vi "Demo Main.vi"() -> ()   [LabVIEW 2022 SP3]
uses:
  Logo.ctl
  C:/Users/Public/OneDrive/Desktop/PMT program/SampleCodeLabView/Kinesis_with_LabVIEW_Examples_LV12 - v3/Thorlabs.MotionControl.Controls.dll
  Kinesis_with_LabVIEW_Examples_LV12 - v3/Thorlabs.MotionControl.Controls.dll
  <vilib>/Utility/file.llb/Write Delimited Spreadsheet (string).vi
  <vilib>/Utility/file.llb/Write Delimited Spreadsheet (I64).vi
  <vilib>/Utility/file.llb/Write Delimited Spreadsheet (DBL).vi
  C:/Users/Public/OneDrive/Desktop/PMT program/SampleCodeLabView/Kinesis_with_LabVIEW_Examples_LV12 - v3/ThorLabs.MotionControl.KCube.DCServoCLI.dll
  Kinesis_with_LabVIEW_Examples_LV12 - v3/ThorLabs.MotionControl.KCube.DCServoCLI.dll
  <vilib>/Analysis/NI_AALBase.lvlib
panel:
  in  "SP 2":i32 caption="Start Position 2 \n Set Data\n(degrees)"
  out "SPD 2":i32 caption="Start Position 2\nRead Data"
  in  "second motor T/F":bool=TRUE
  out "PC 2":i32 caption="Current \nPosition 2"
  in  "Motor Controller\nSerialNumber 2":string="27260805"
  in  "KCubeDCServoControl 2":refnum<k24>(container)
  out "Polar Plot":picture
  in  "Wait to Start (ms)":i32
  in  "Laser Power (mW)":string="sample"
  in  "Sample Name":string="sample"
  in  "Save All Gate Data":bool
  out "ESD":i32=10000 caption="Steps\nAdded/Removed"
  in  "ES":i32 caption="Add /Remove \nSteps"
  out "Sweep Graph":u32[](graph)
  out "SM":i32 caption="Sweep\nMean"
  out "SN":i32 caption="Current Sweep Iteration"
  out "SND":i32 caption="Total No. of Sweeps"
  in  "Auto-Sweep":bool
  in  "P8":bool
  out "PC":i32 caption="Current \nPosition"
  out "WTD":i32=10000 caption="Wait Time (ms)\nRead Data"
  out "EPD":i32 caption="End Position\nRead Data"
  out "SPD":i32 caption="Start Position\nRead Data"
  out "SSD":i32 caption="Step Size\nRead Data"
  in  "SP":i32 caption="Start Position (degrees)\n Set Data"
  in  "WT":i32=5000 caption="Wait Time (ms)\n Set Data"
  in  "EP":i32 caption="End Position (degrees)\n Set Data"
  in  "P7":bool
  in  "SS":i32=10 caption="Step Size (degrees)\nSet Data"
  in  "Motor Controller\nSerialNumber":string="27261255"
  in  "KCubeDCServoControl":refnum<k24>(container)
  in  "Export":bool
  out "DB":u32[](array[numeric])
  out "OVL":bool caption="LED ON : Over Rang Data"
  out "OLD":i32
  out "GN":i32 caption="Gate Number"
  in  "Correction":bool=TRUE
  in  "Logo":T1
  out "Graph":u32[](graph)
  in  "Stop":bool
  in  "Start":bool
  in  "P6":bool
  out "RND":i32 caption="Read Number\nRead Data"
  in  "P5":bool
  in  "RN":i32=40 caption="Read Number\nSet Data"
  out "PowerD":i32 caption="Power\nRead Data"
  out "ITD":i32 caption="Internal Time\nRead Data"
  in  "P4":bool
  in  "P3":bool
  in  "IT":i32=100 caption="Internal Time\nSet Data"
  in  "P2":bool
  out "Handle Number":i32
  in  "P1":bool caption="Switch\nPower OFF/Power ON"
  in  "EXIT":bool
  # "pmt serial: 30430219"
  # "can't change after running. exit to change"
  # "note: If you change angle between linear polarized light and half-wave plate by theta, the \npolarization after the wave plate is changed by twice theta. The code doesn't account for this.\nThis means we really need to go only to 180degrees, because at that point we have rotated the polarization by 360deg."
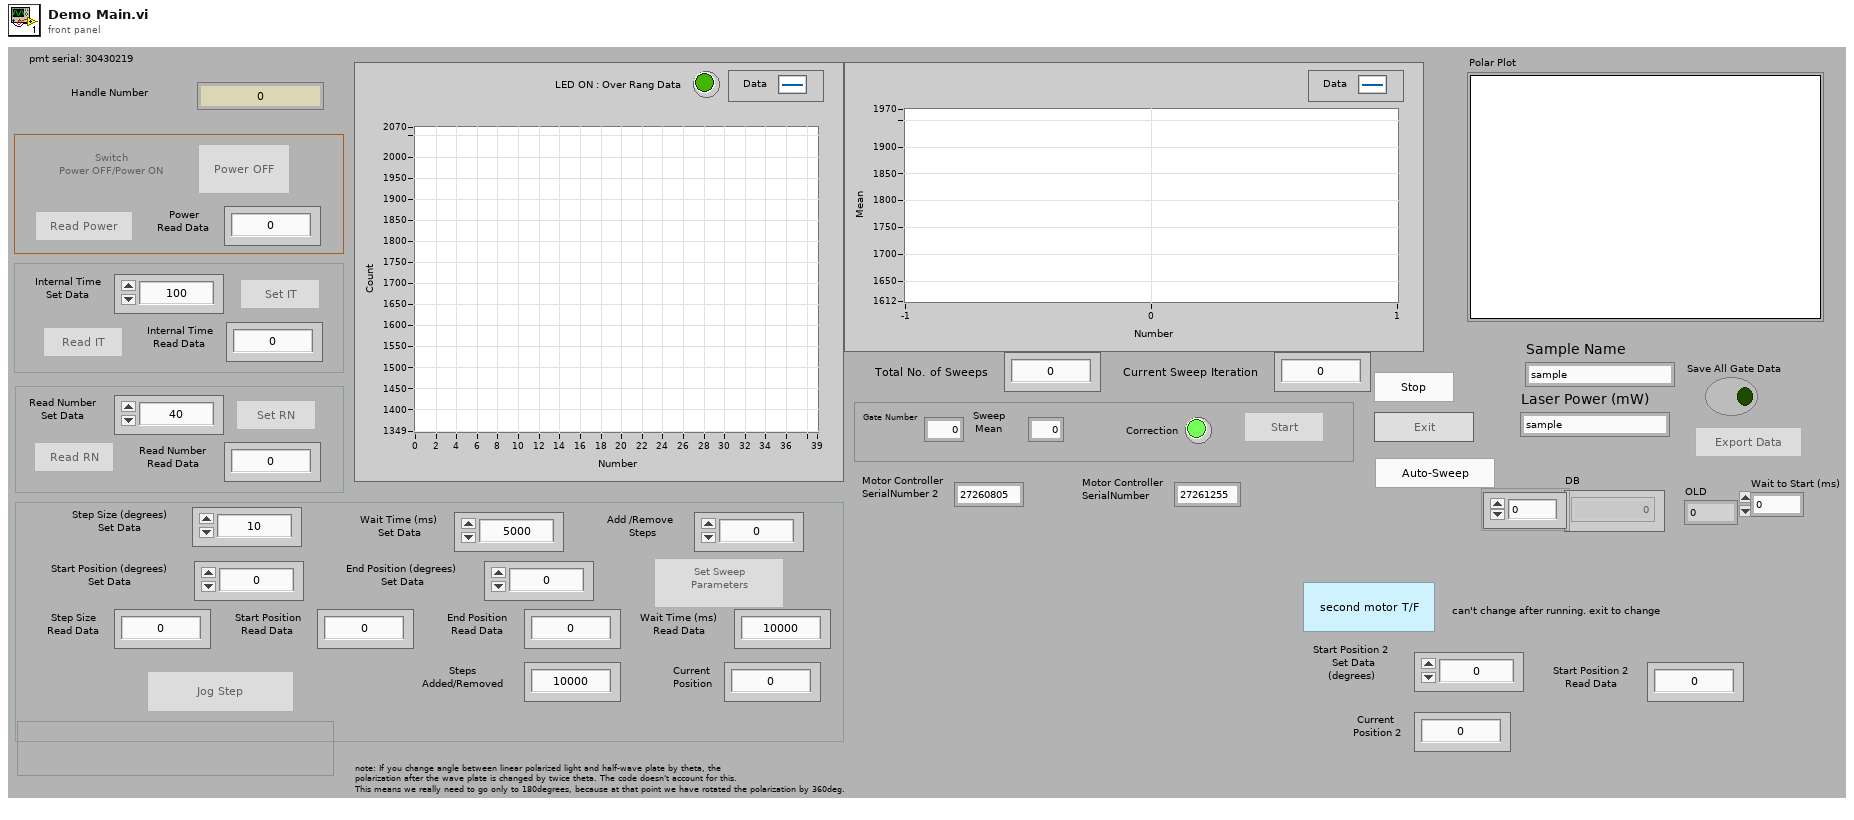
[diagram p1: front panel]
types:
  T1 = typedef "Logo.ctl" = bool
  T2 = enum8{"Enabled", "Disabled", "Disabled and Grayed Out"}
  T3 = typedef "LVBoundsTypeDef.ctl" = cluster{"Width":u32, "Height":u32}
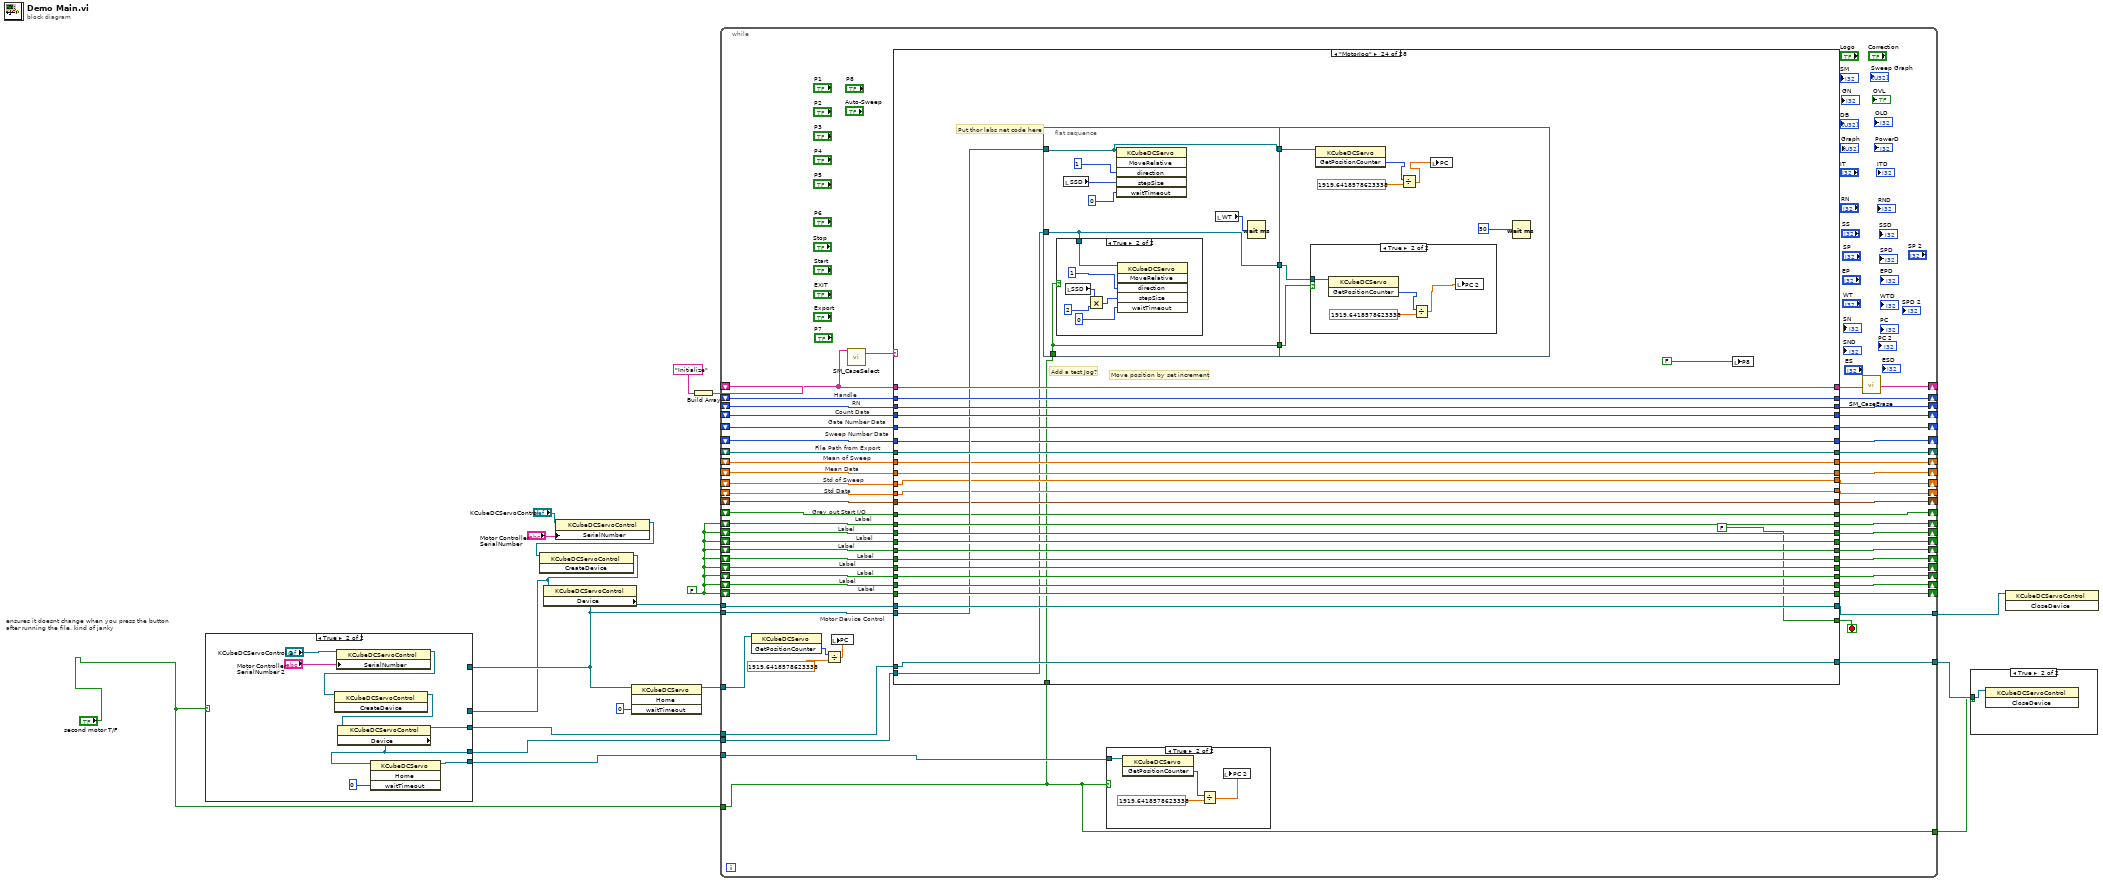
[diagram p0: block diagram]
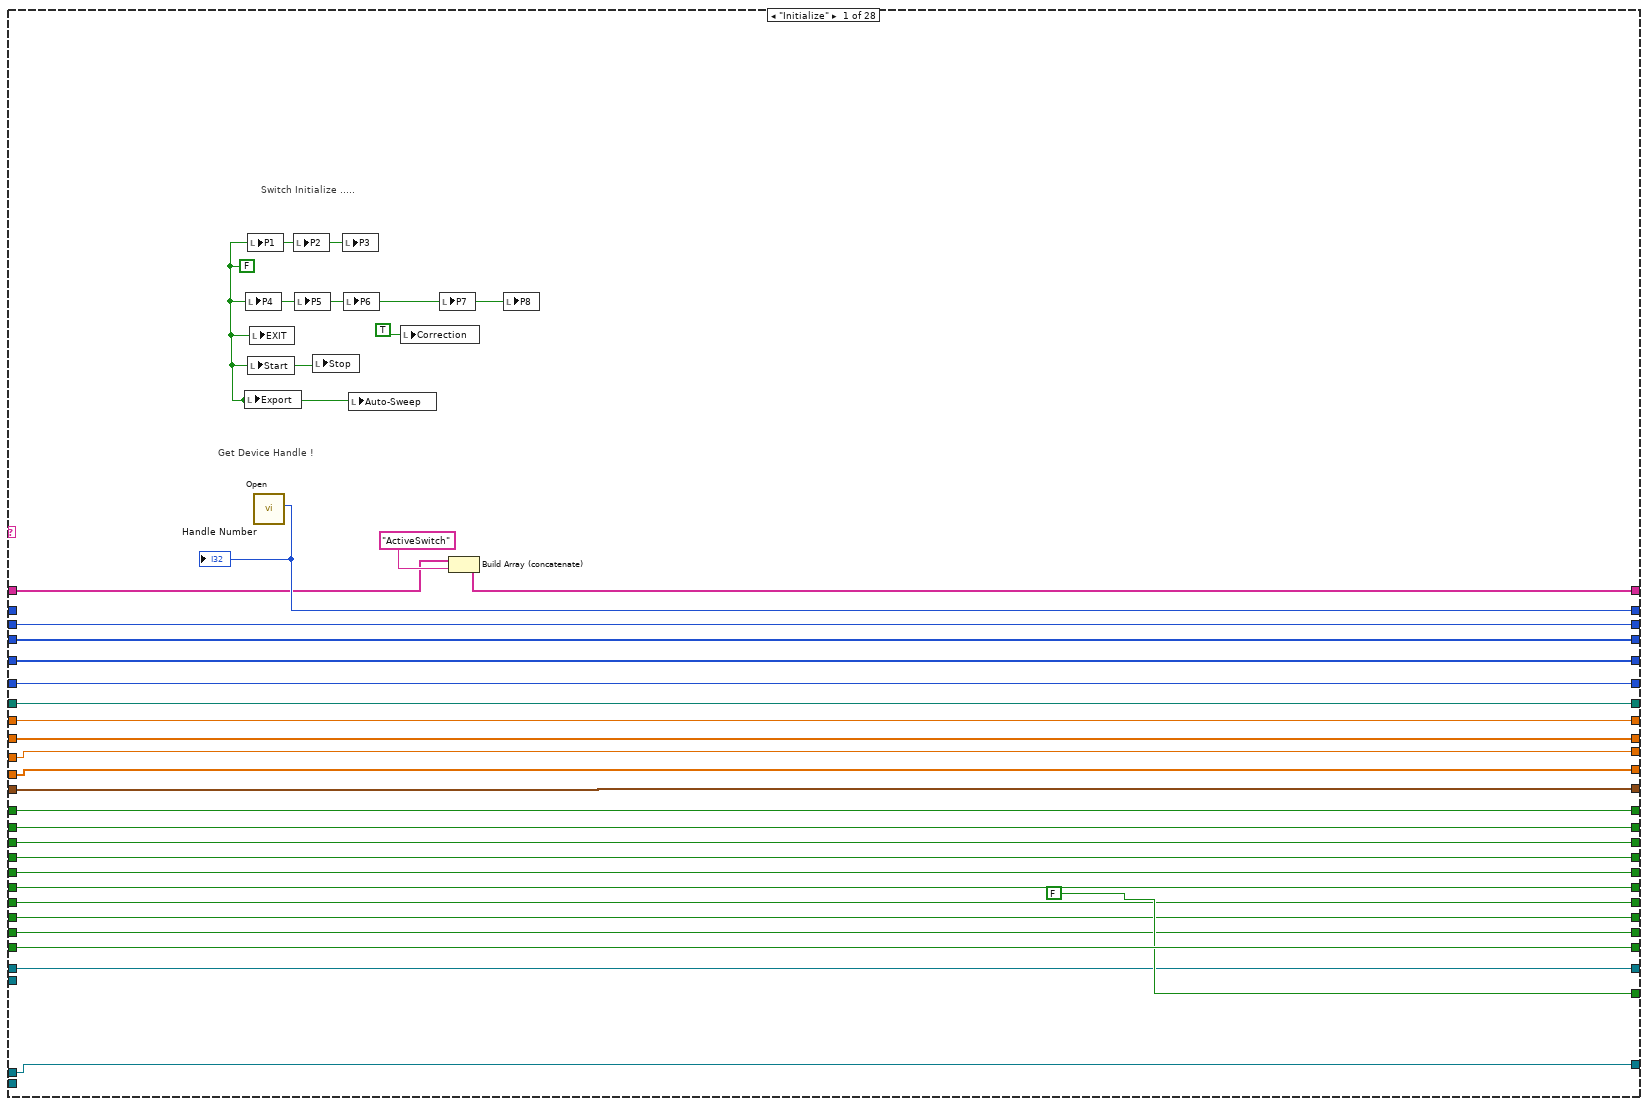
[diagram p5: hidden frame]
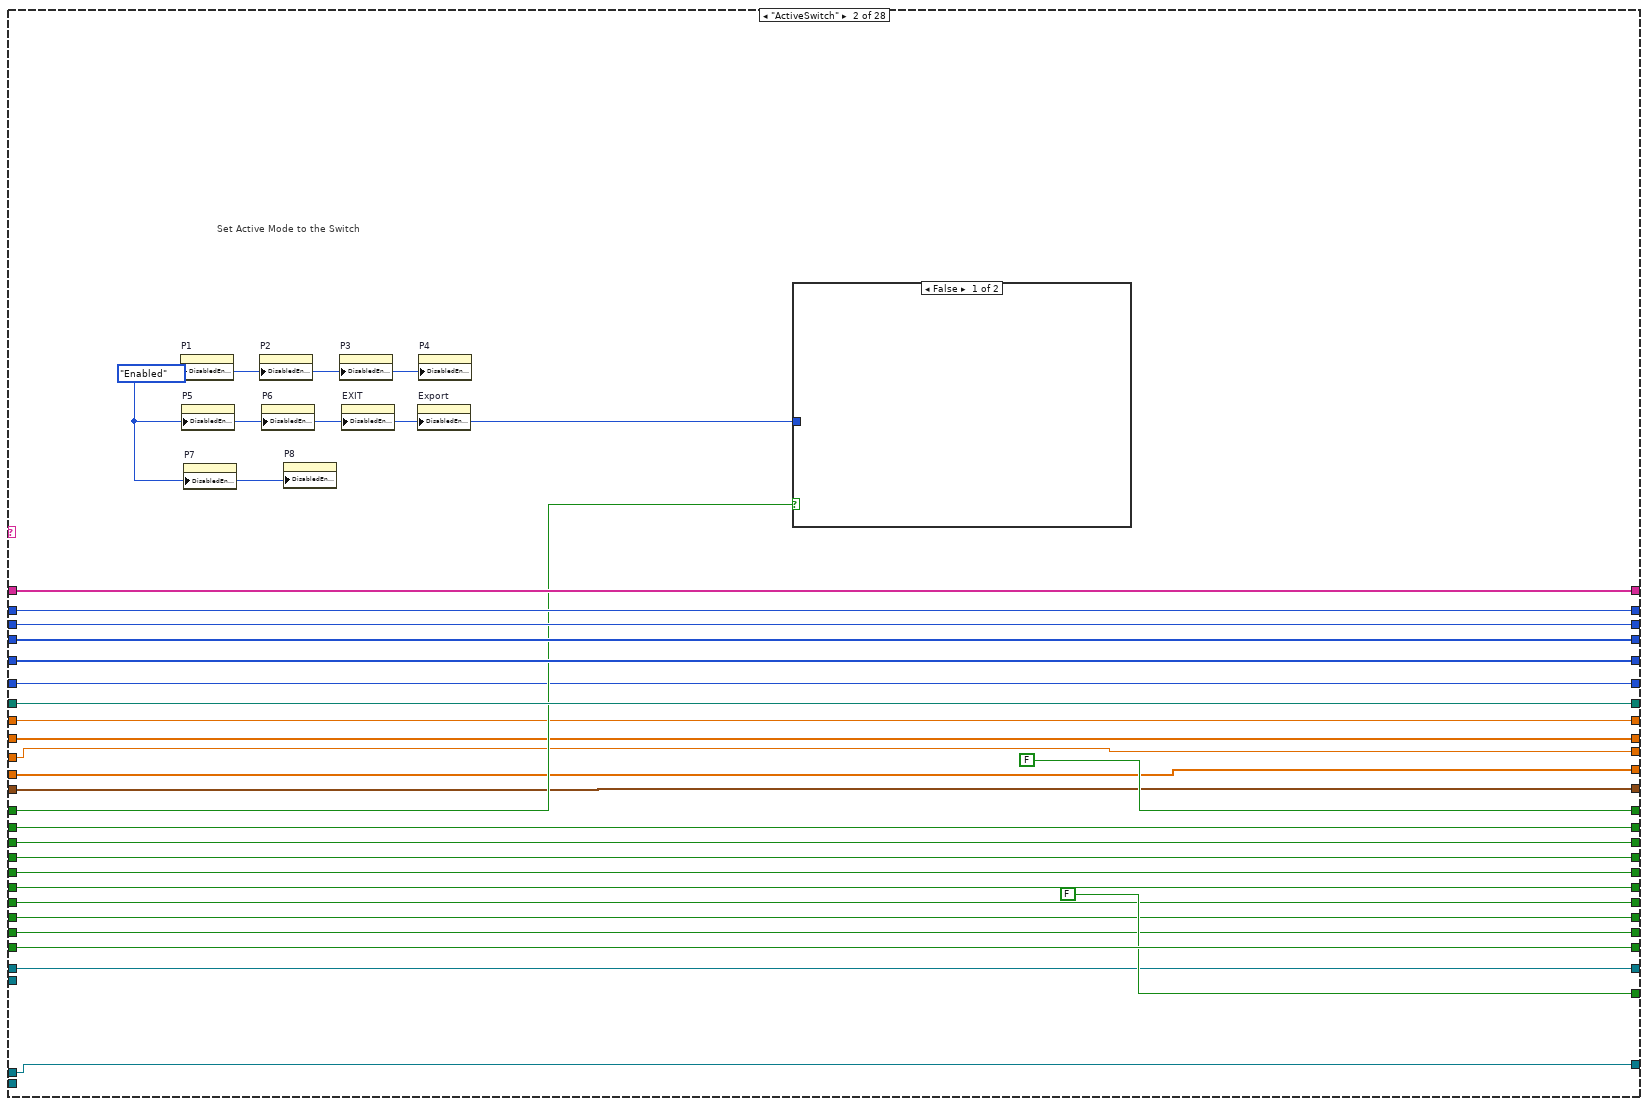
[diagram p6: hidden frame]
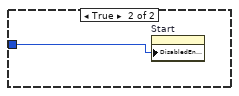
[diagram p7: hidden frame]
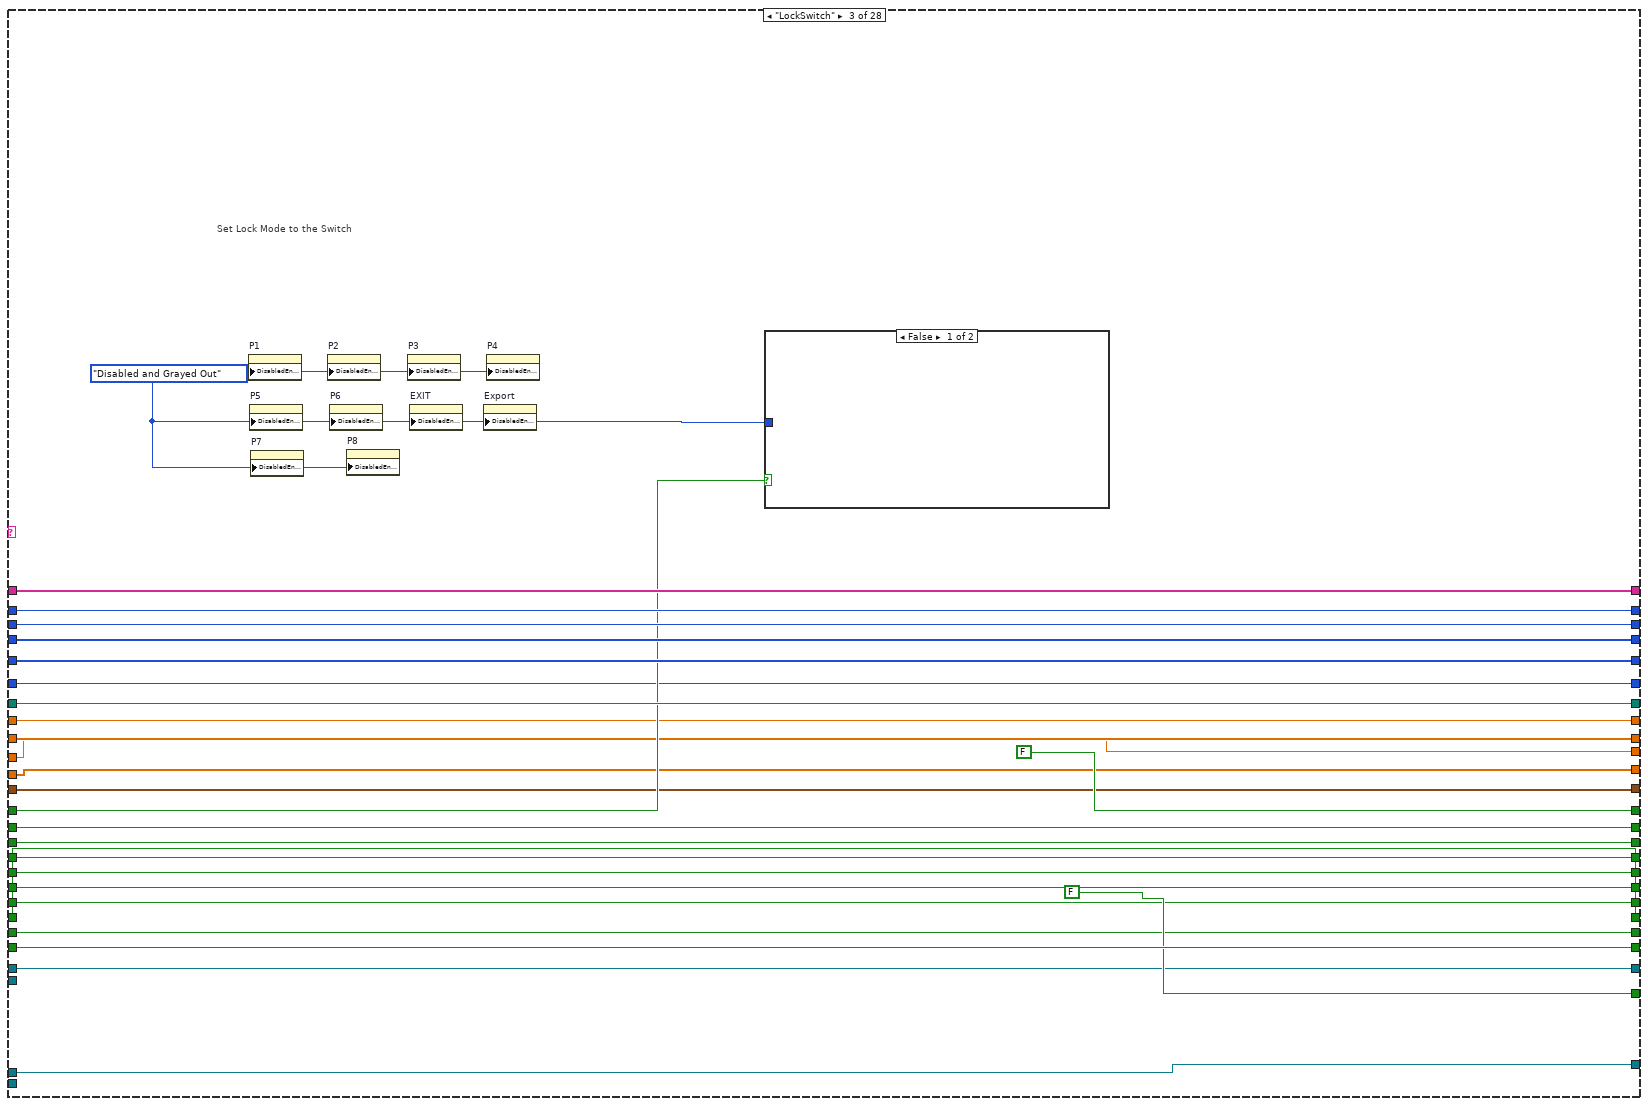
[diagram p8: hidden frame]
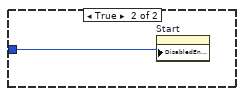
[diagram p9: hidden frame]
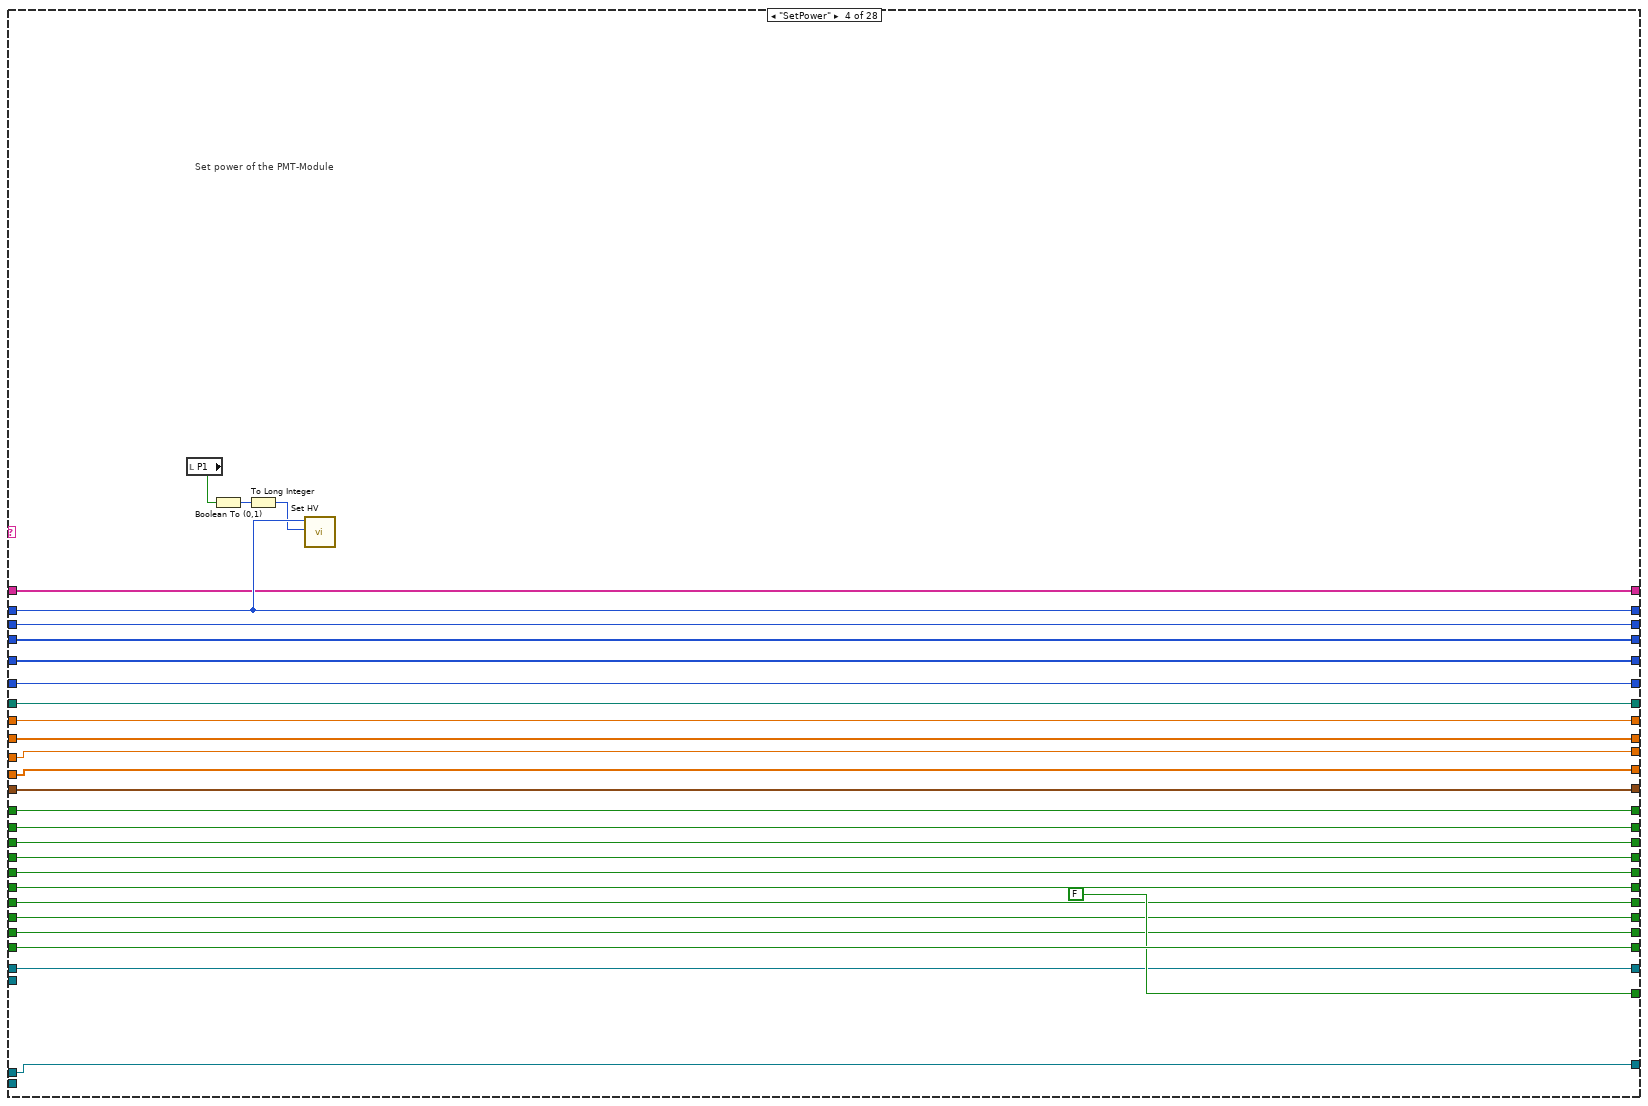
[diagram p10: hidden frame]
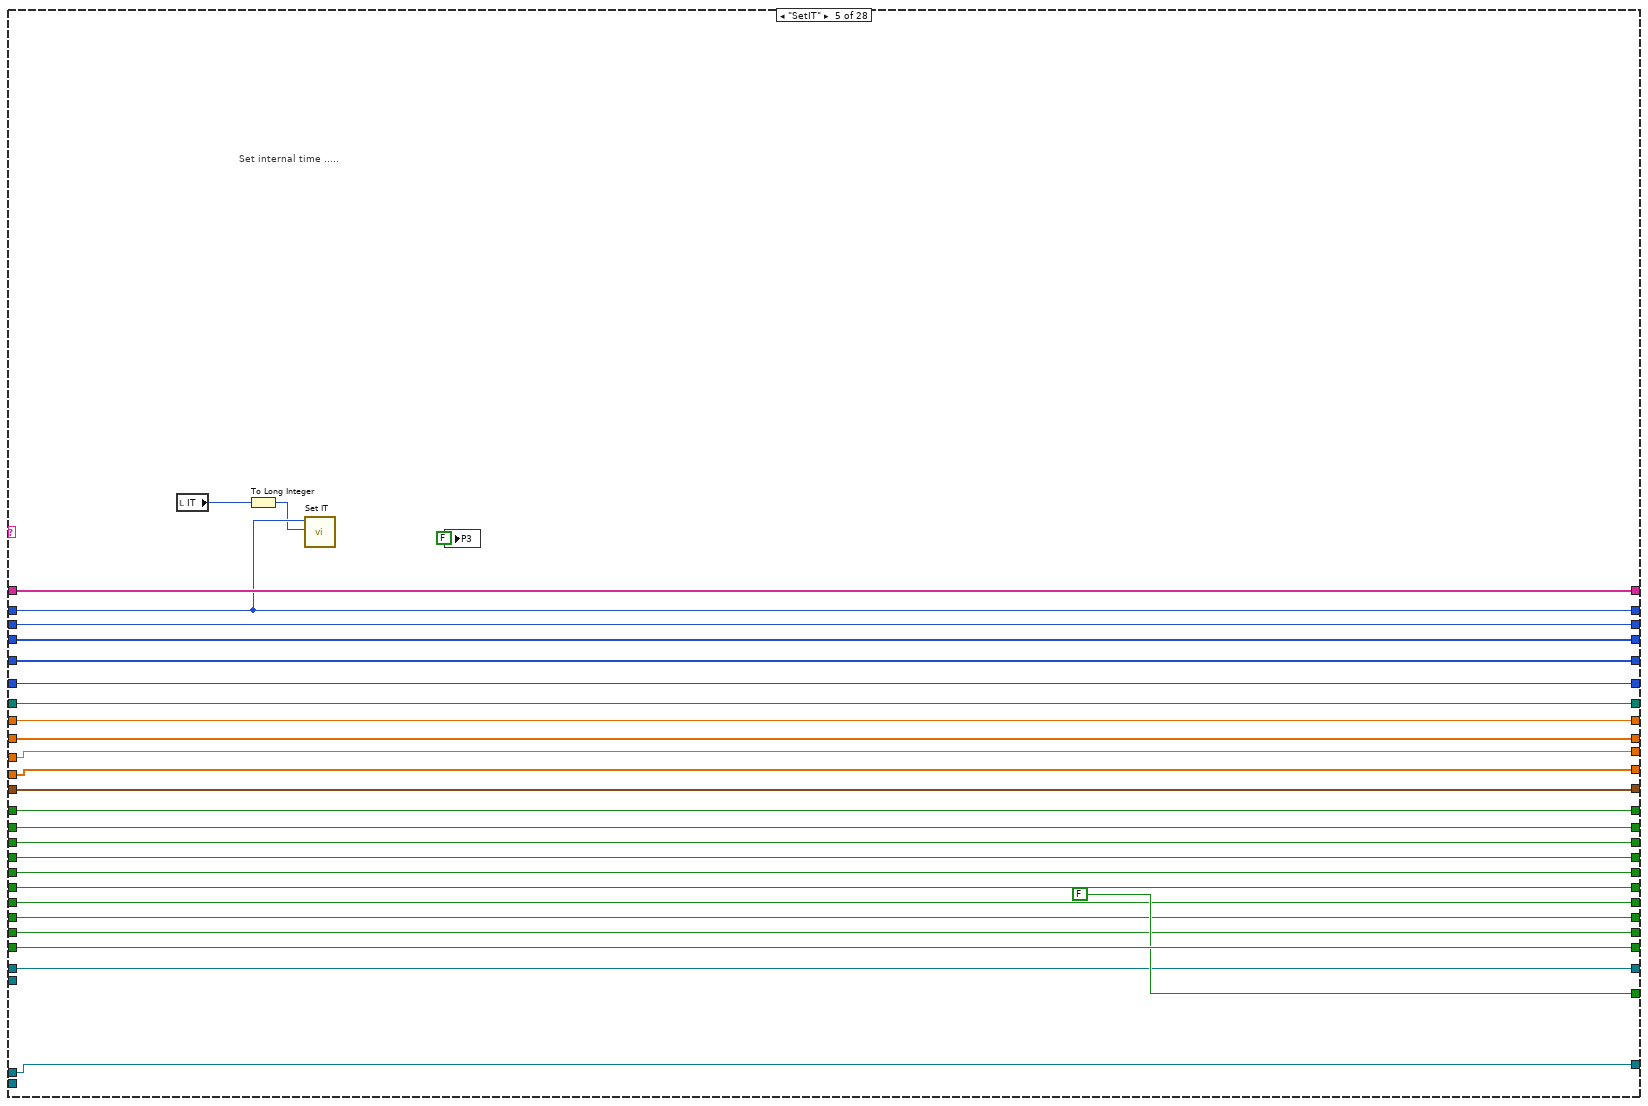
[diagram p11: hidden frame]
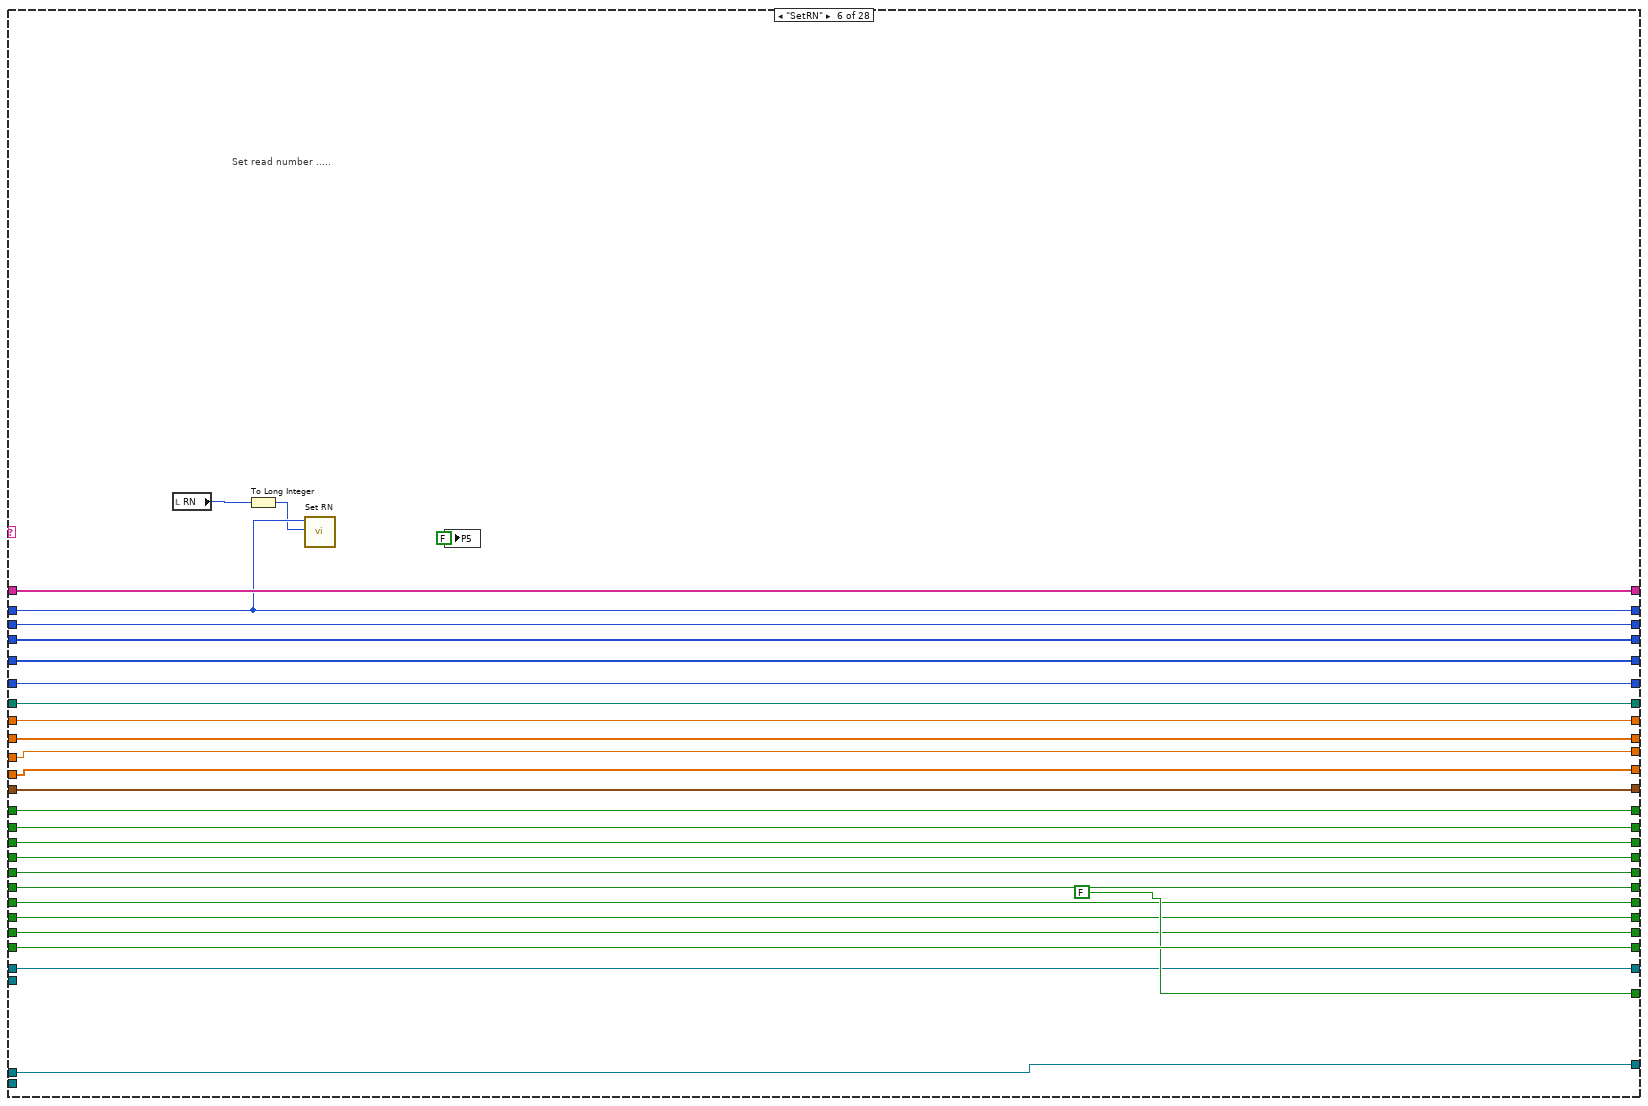
[diagram p12: hidden frame]
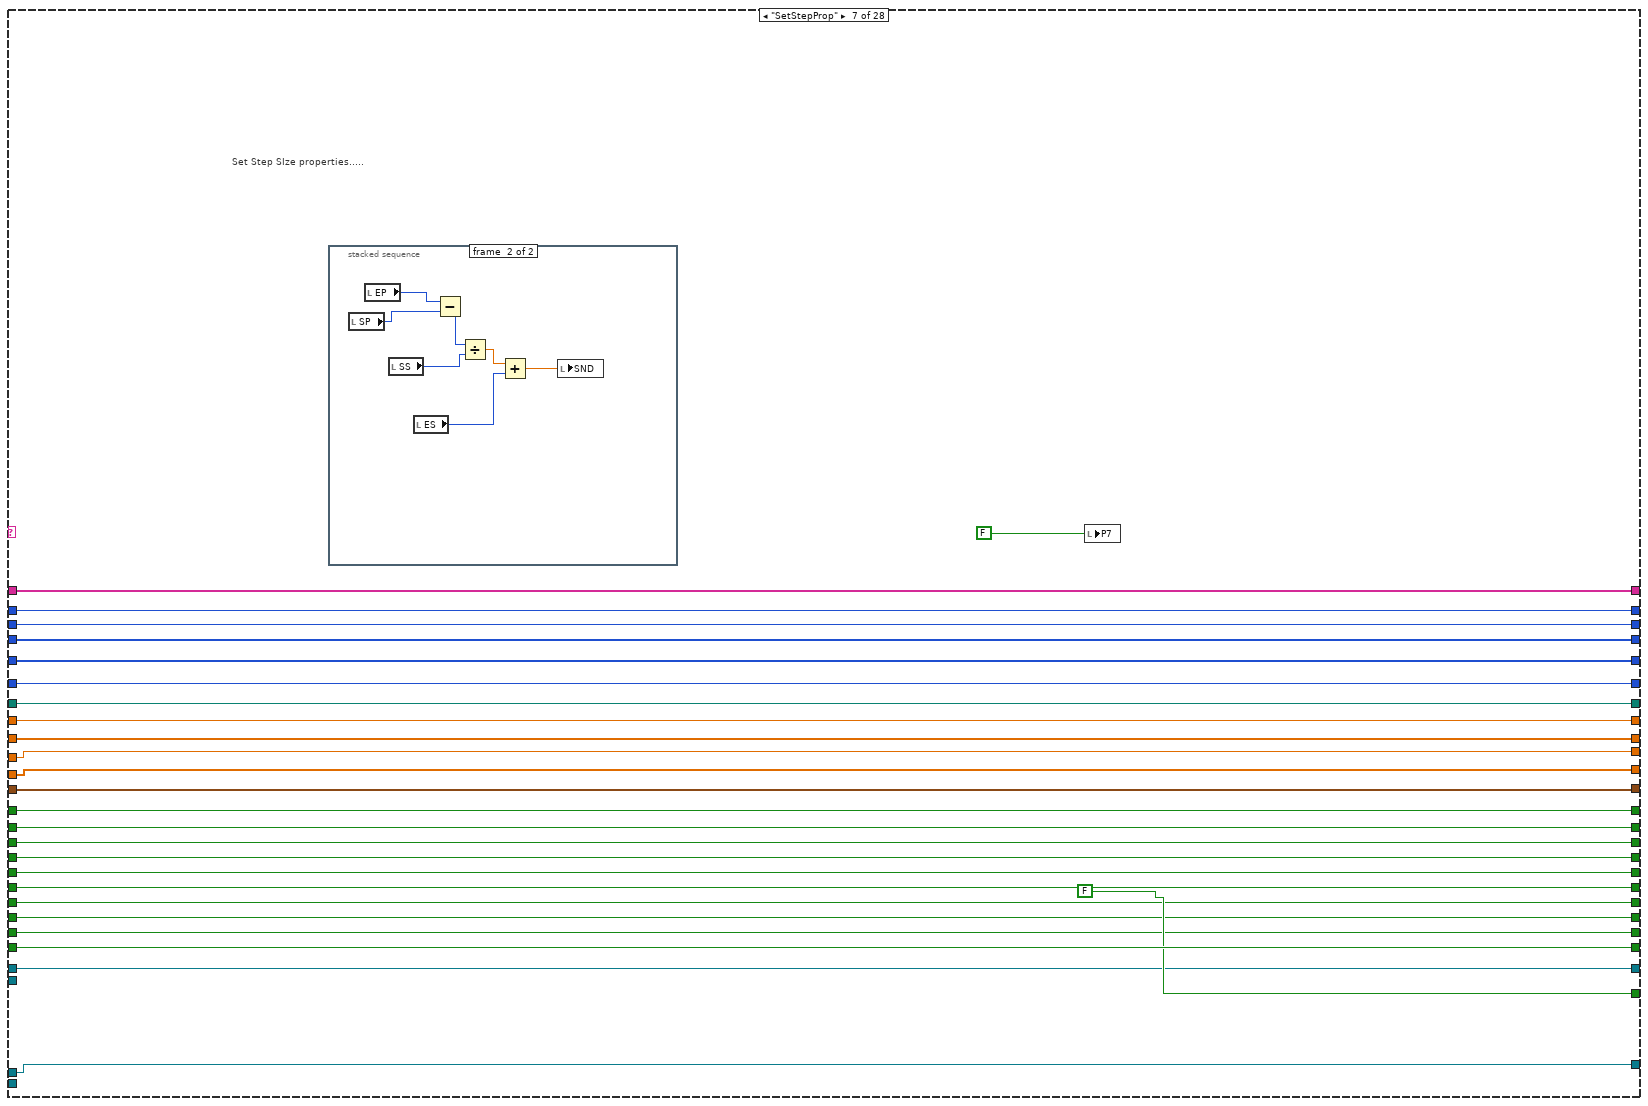
[diagram p13: hidden frame]
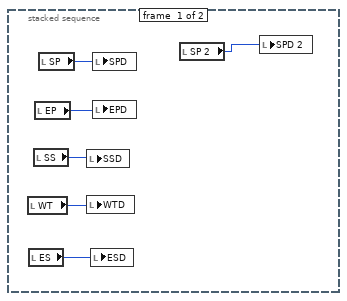
[diagram p14: hidden frame]
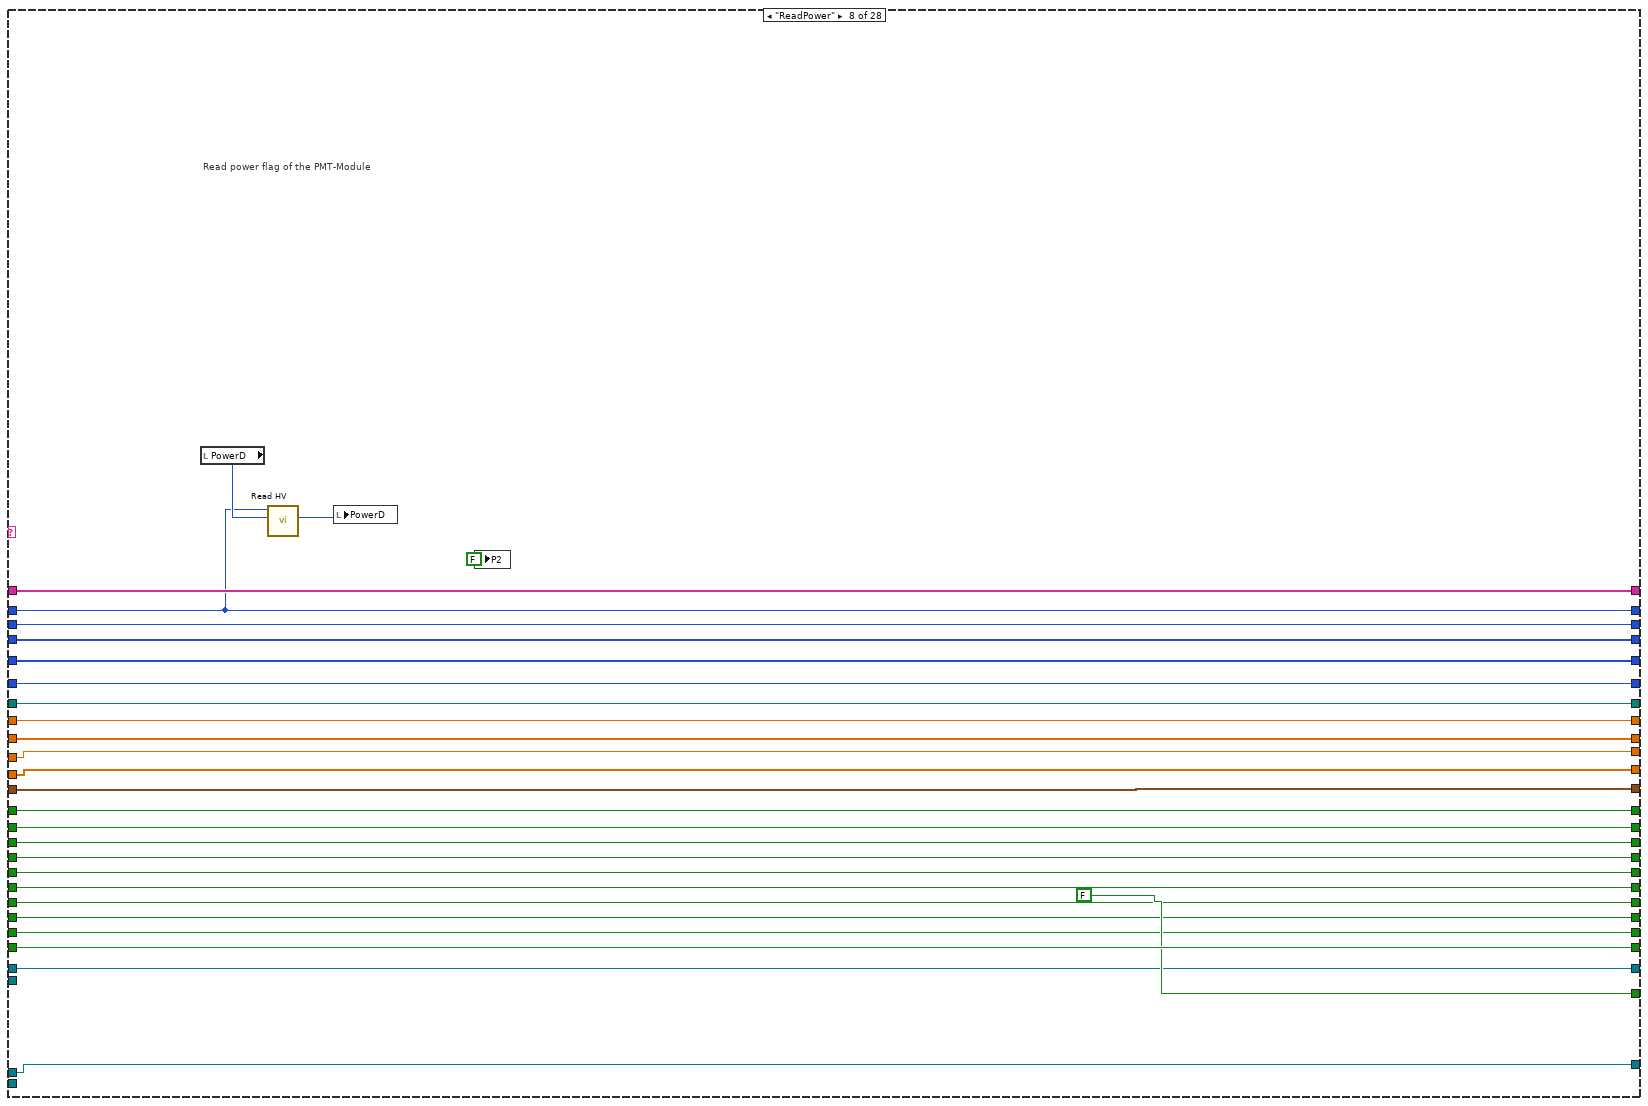
[diagram p15: hidden frame]
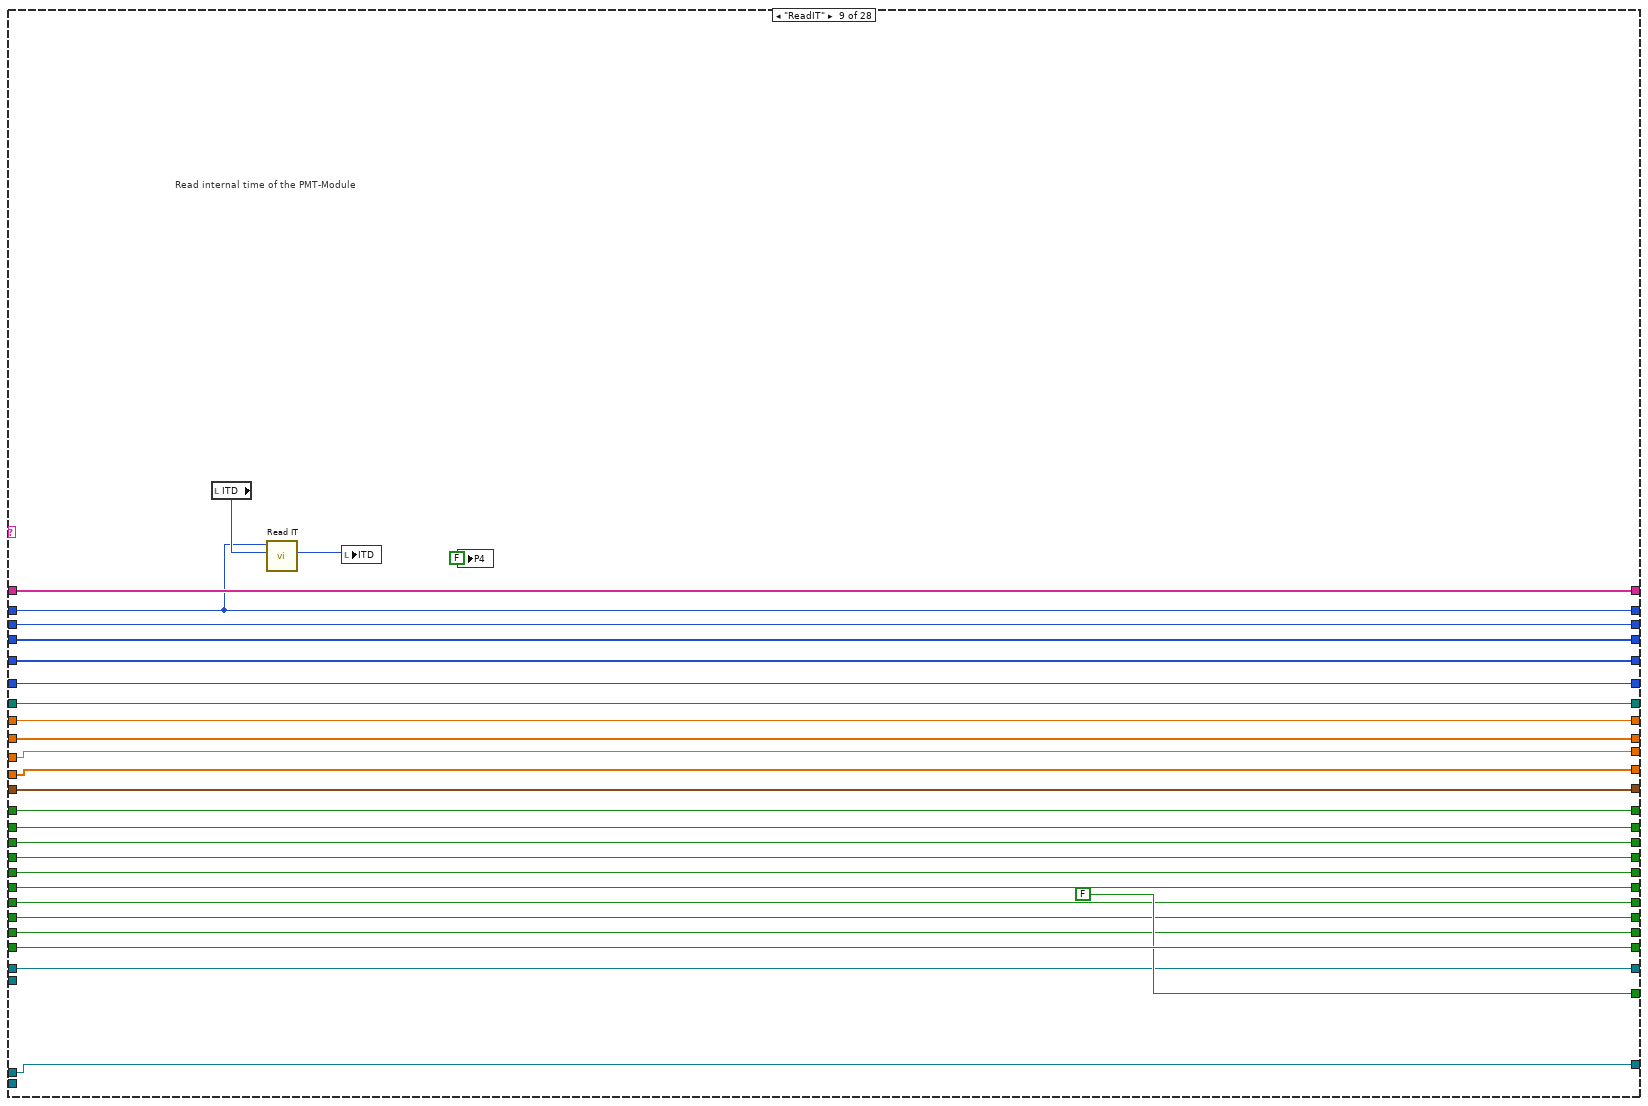
[diagram p16: hidden frame]
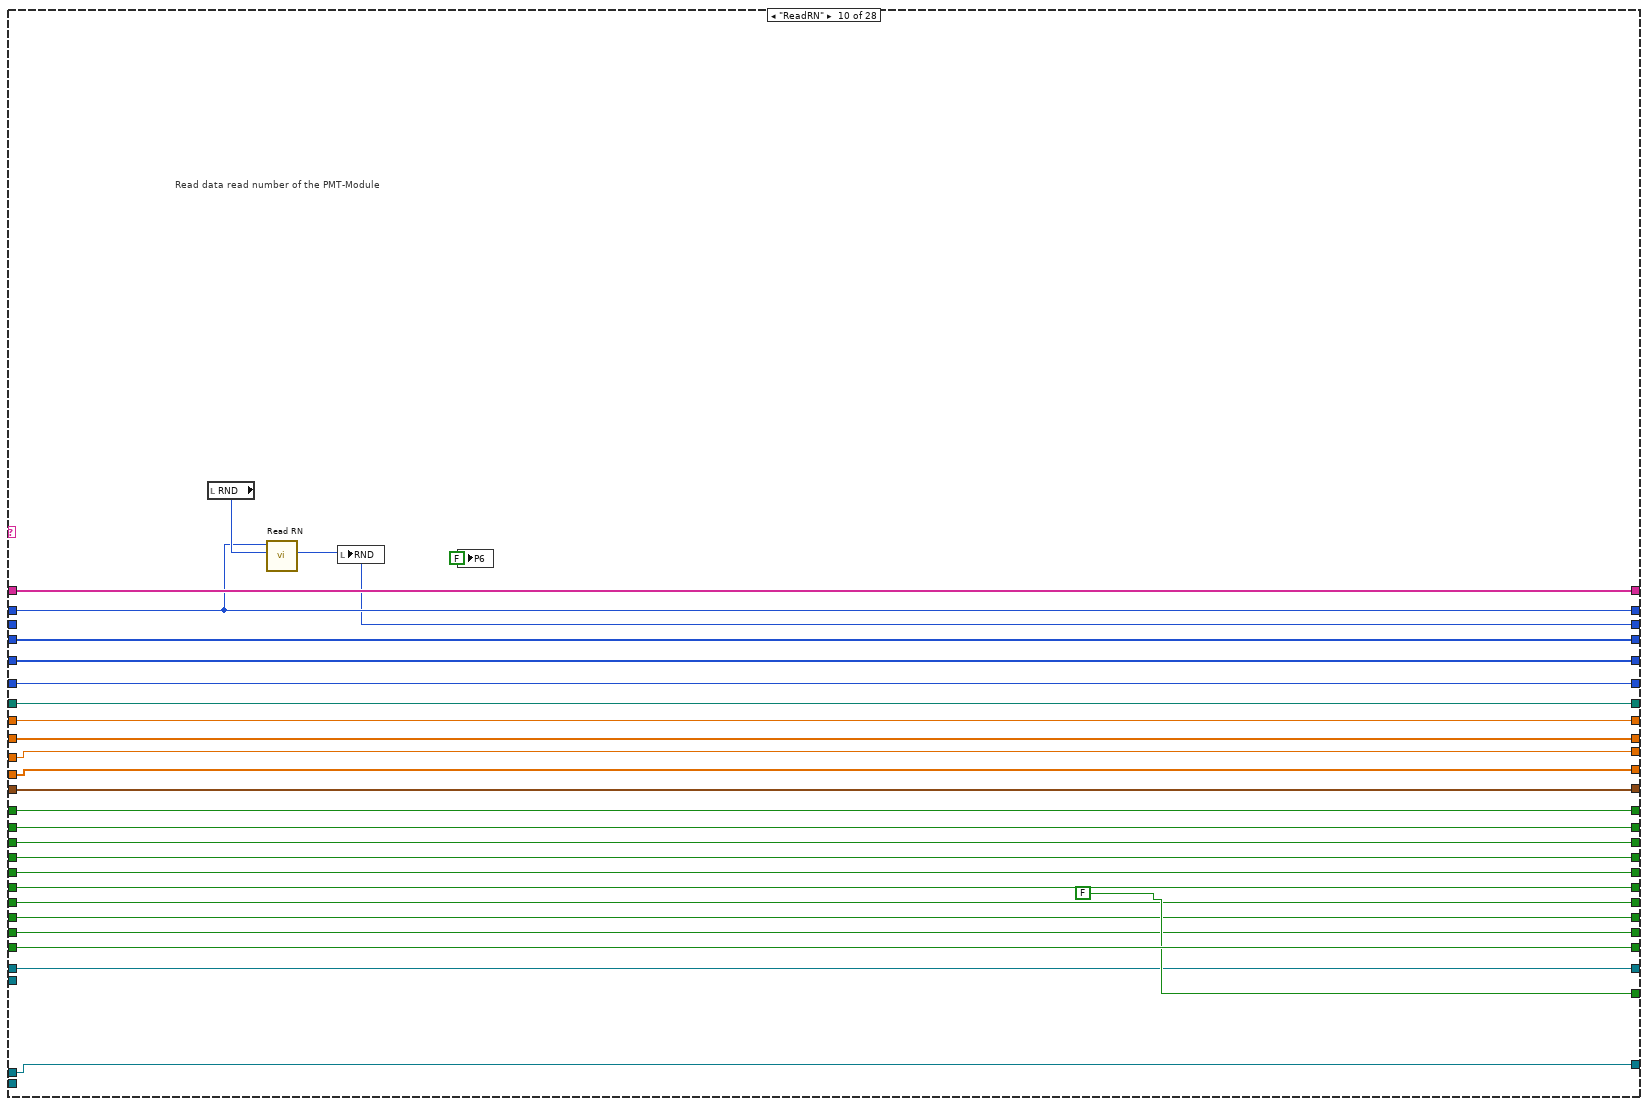
[diagram p17: hidden frame]
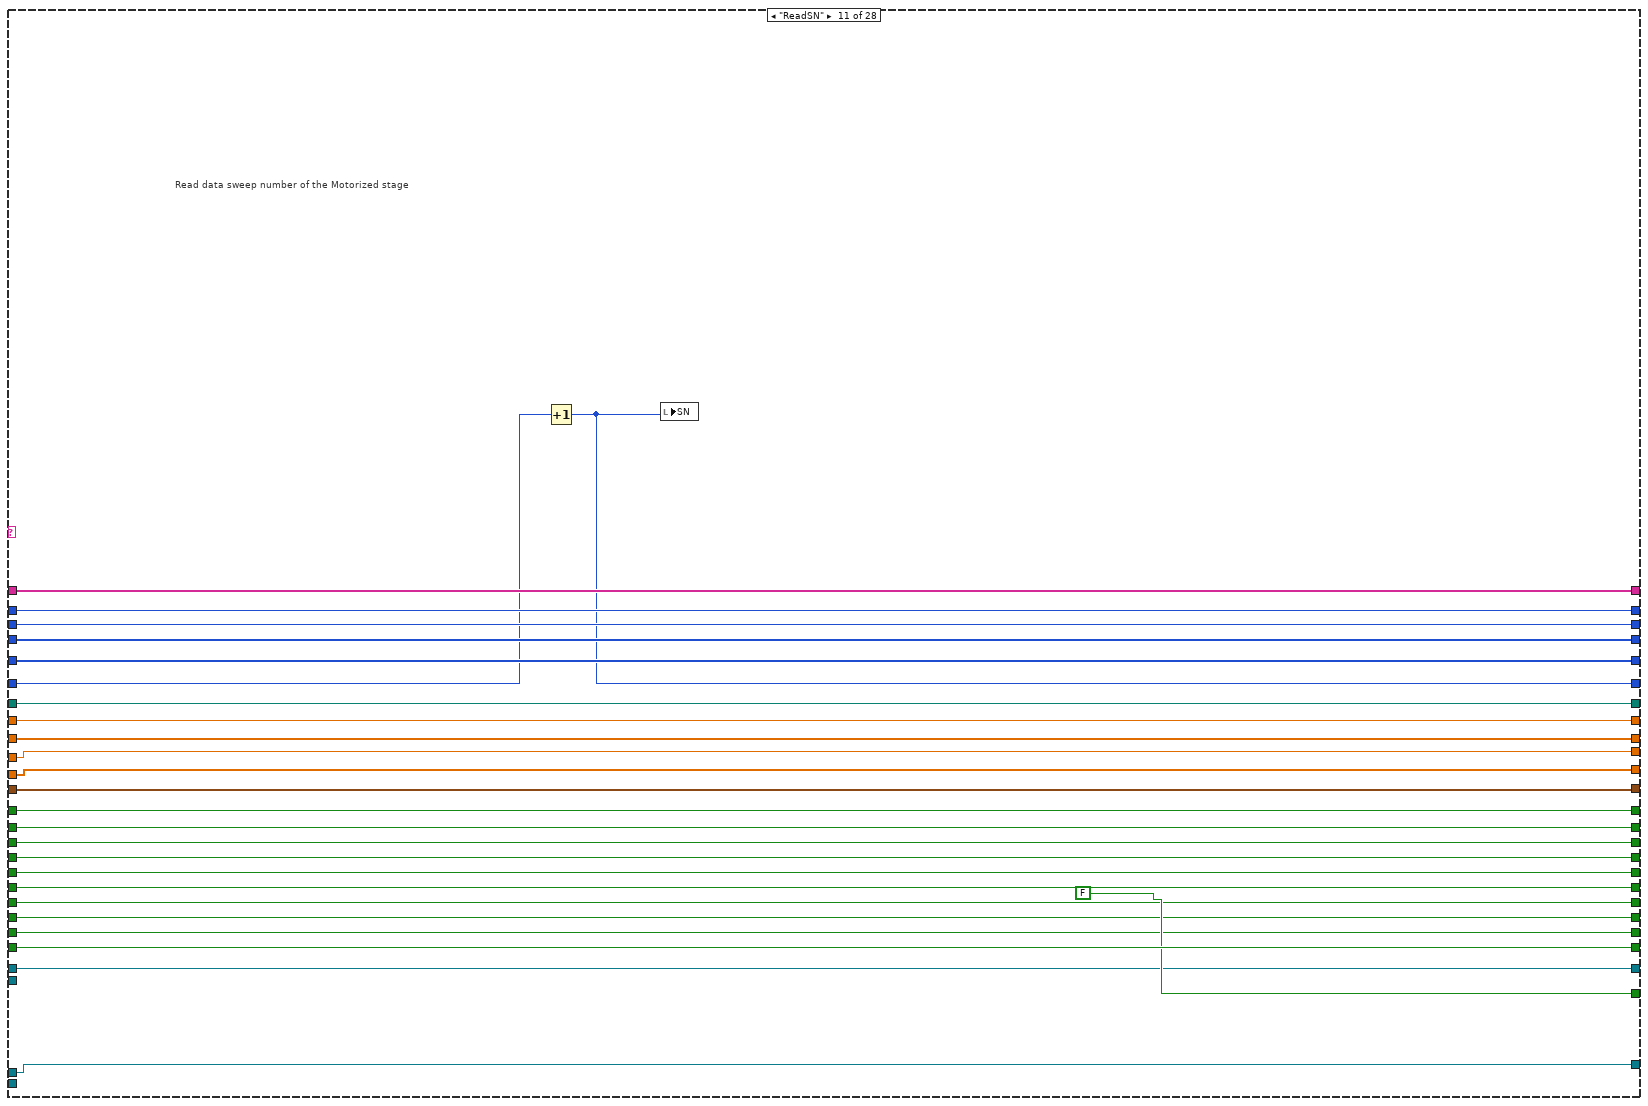
[diagram p18: hidden frame]
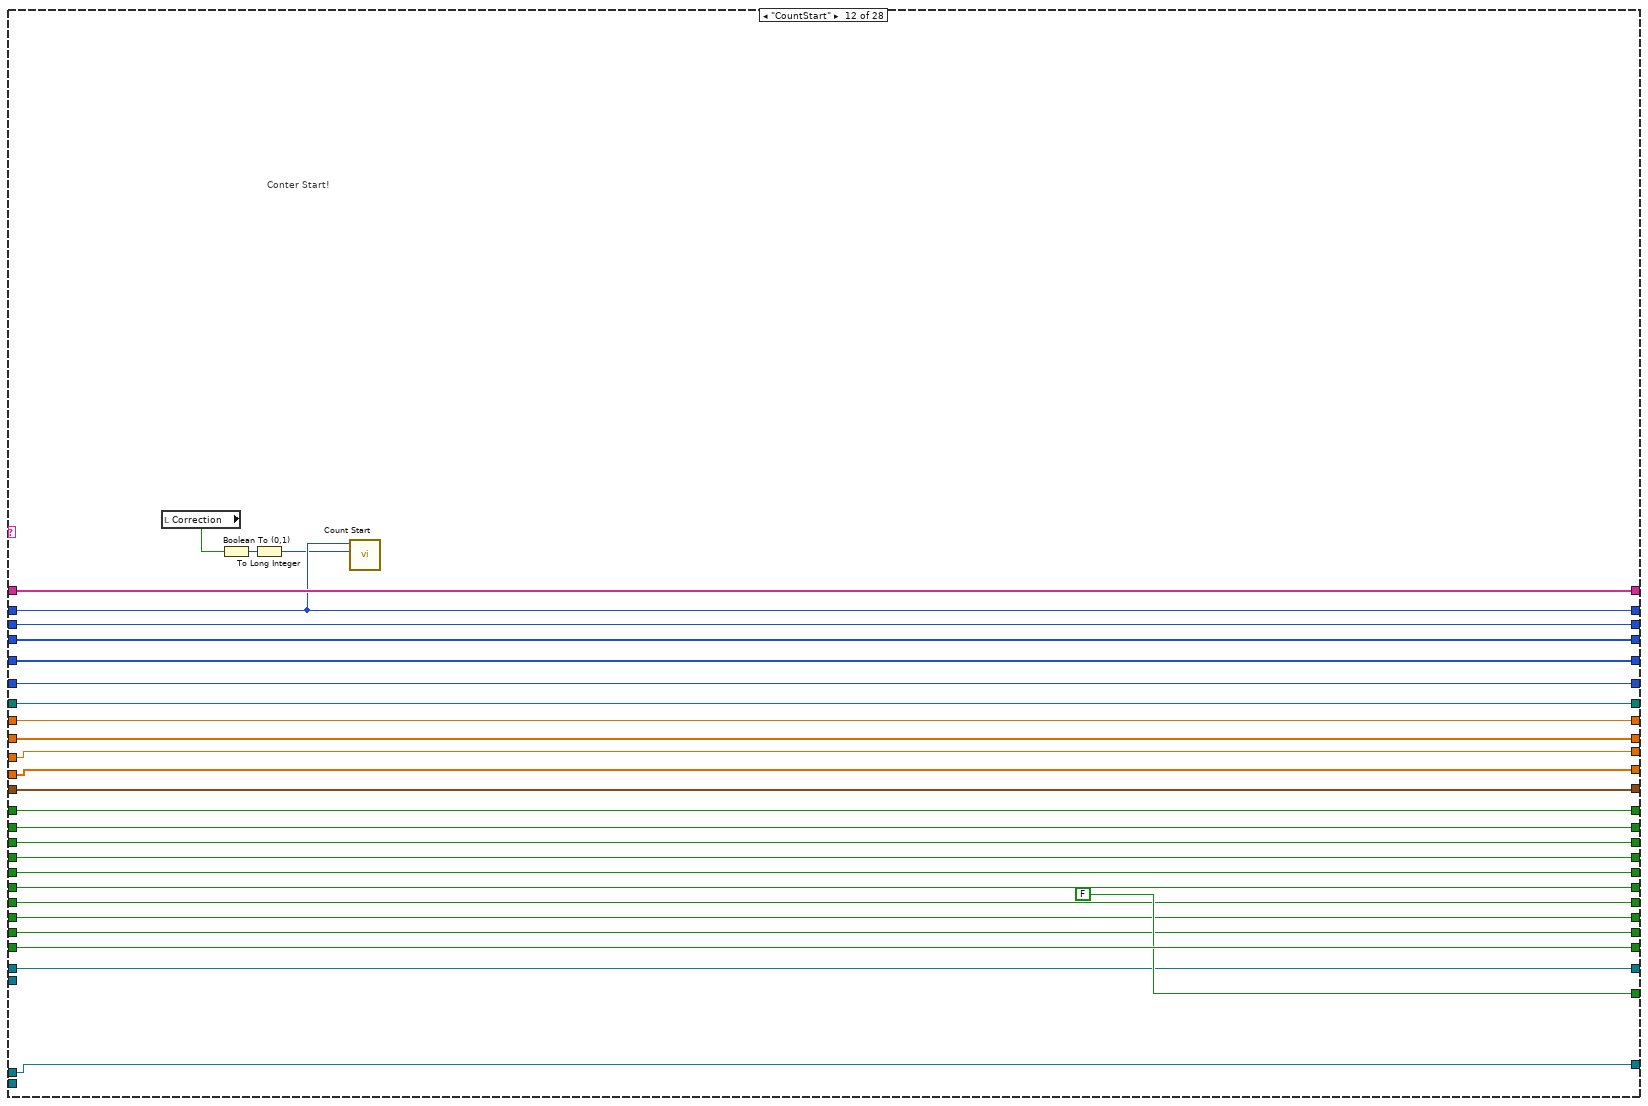
[diagram p19: hidden frame]
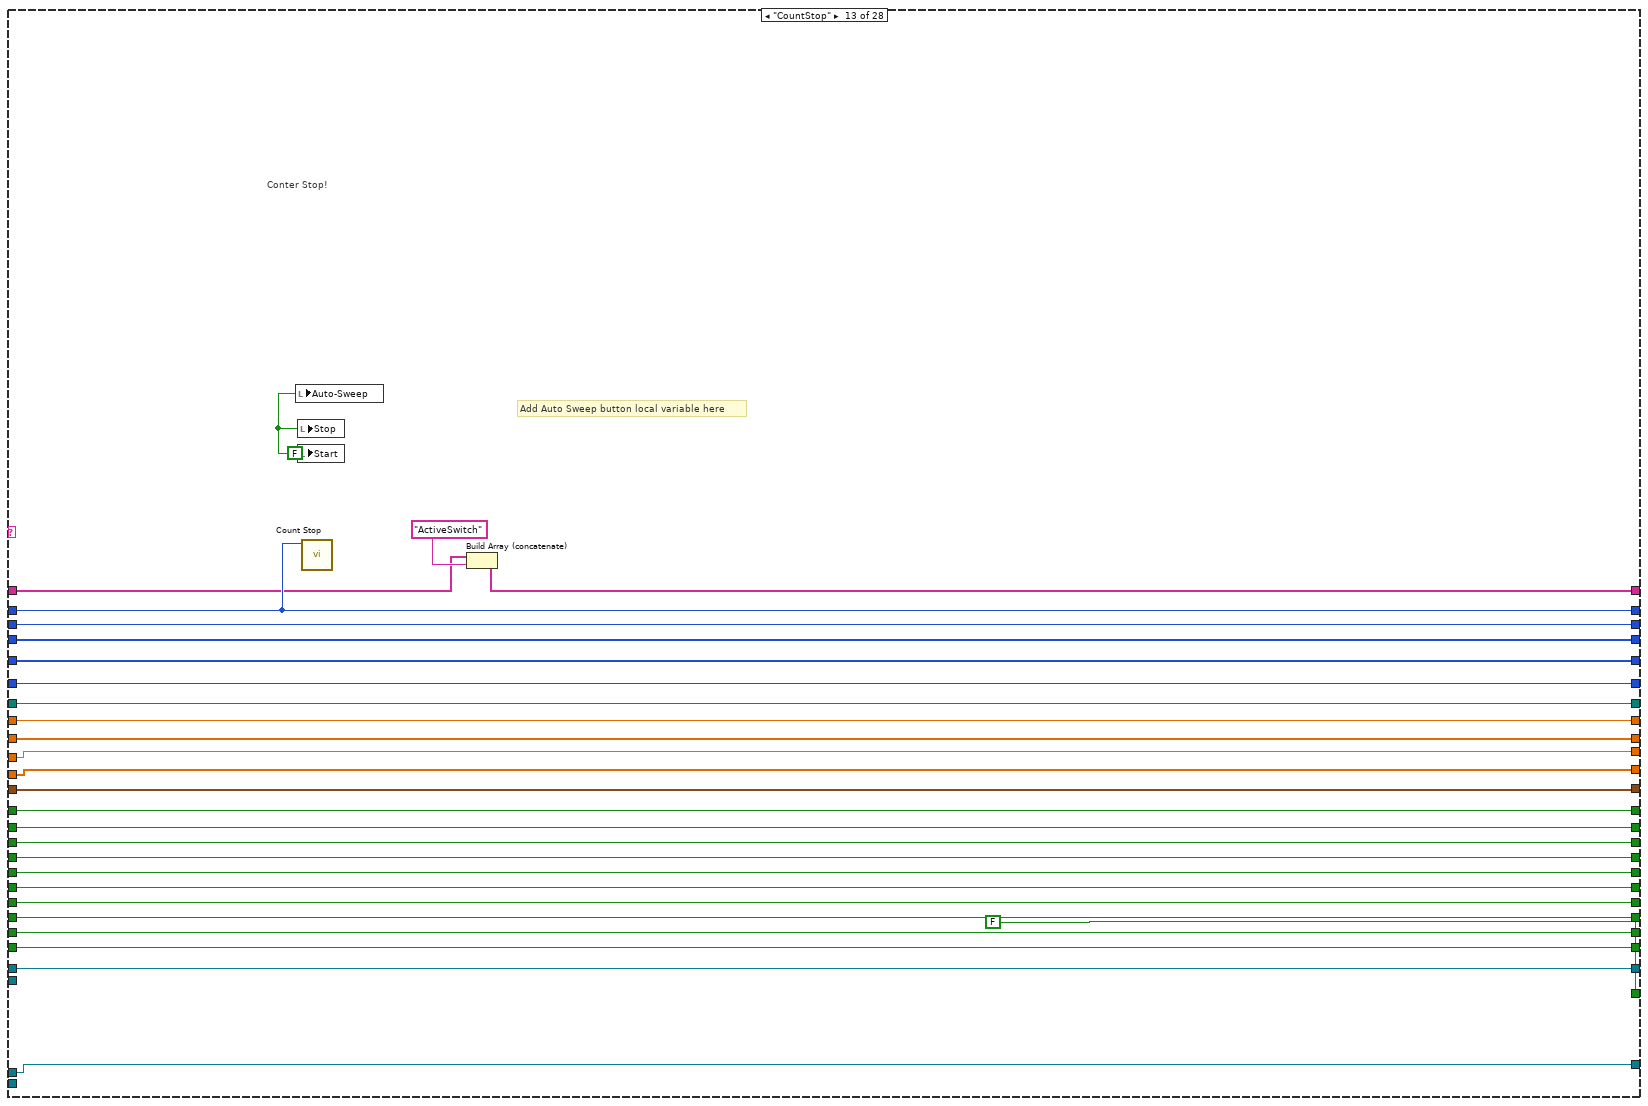
[diagram p20: hidden frame]
diagram:
  w16 = FALSE
  # "ensures it doesnt change when you press the button \nafter running the file. kind of janky"
  n1 = property class="KCubeDCServoControl"(reference="KCubeDCServoControl", "SerialNumber"="Motor Controller\nSerialNumber") -> (reference out=w15:refnum<k24>)  [unwired: 1 in, 1 out]
  n2 = invoke class="KCubeDCServoControl" method="CreateDevice"(reference=w15) -> (reference out=w3:refnum<k24>)  [unwired: 2 in, 2 out]
  n3 = property class="KCubeDCServoControl"(reference=w3) -> (reference out=w12:refnum<k24>, "Device"=w4:refnum<k24>)  [unwired: 1 in, 1 out]
  n4 = case shown="True" "second motor T/F" {
    tunnel: [w19 w23] -> w8
    tunnel: [w19 w22] -> w7
    tunnel: [w20 w21] -> w6
    tunnel: w4 -> [w19 _]
    tunnel: w3 -> [w20 _]
    frame False {
      # "just connect to the first one. it won't be sused"
    }
    frame True {
      n5 = property class="KCubeDCServoControl"(reference="KCubeDCServoControl 2", "SerialNumber"="Motor Controller\nSerialNumber 2") -> (reference out=w28:refnum<k24>)  [unwired: 1 in, 1 out]
      n6 = invoke class="KCubeDCServoControl" method="CreateDevice"(reference=w28) -> (reference out=w25:refnum<k24>)  [unwired: 2 in, 2 out]
      n7 = property class="KCubeDCServoControl"(reference=w25) -> (reference out=w21:refnum<k24>, "Device"=w22:refnum<k24>)  [unwired: 1 in, 1 out]
      n8 = invoke class="KCubeDCServo" method="Home"(reference=w22, "waitTimeout"=0) -> (reference out=w23:refnum<k24>)  [unwired: 2 in, 3 out]
    }
  }
  n9 = invoke class="KCubeDCServo" method="Home"(reference=w4, "waitTimeout"=0) -> (reference out=w10:refnum<k24>)  [unwired: 2 in, 3 out]
  n10 = Build Array("Initialize") -> (w17:string[])
  n11 = while {
    shift-right: [w70] -> _
    shift-left: w16 -> [w71]
    shift-right: [w72] -> _
    shift-left: w16 -> [w73]
    shift-right: [w74] -> _
    shift-left: w16 -> [w75]
    shift-right: [w76] -> _
    shift-left: w16 -> [w77]
    shift-right: [w78] -> _
    shift-left: _ -> [w79]
    shift-right: [w80] -> _
    shift-left: _ -> [w81]
    shift-right: [w82] -> _
    shift-left: _ -> [w83]
    shift-right: [w68] -> _
    shift-left: w16 -> [w69]
    shift-right: [w86] -> _
    shift-left: w16 -> [w87]
    shift-right: [w65] -> _
    shift-left: w17 -> [w84]
    shift-right: [w63] -> _
    shift-left: w16 -> [w64]
    shift-right: [w61] -> _
    shift-left: w16 -> [w62]
    shift-right: [w60] -> _
    shift-left: w16 -> [w59]
    tunnel: w12 -> [w56]
    tunnel: [w55] -> w13
    shift-right: [w58] -> _
    shift-left: _ -> [w57]
    tunnel: w4 -> [w54]
    shift-right: [w53] -> _
    shift-left: _ -> [w52]
    shift-right: [w51] -> _
    shift-left: _ -> [w50]
    tunnel: w10 -> [w49]
    shift-right: [w47] -> _
    shift-left: _ -> [w48]
    shift-right: [w46] -> _
    shift-left: _ -> [w45]
    shift-right: [w44] -> _
    shift-left: _ -> [w43]
    shift-right: [w39] -> _
    shift-left: _ -> [w40]
    shift-right: [w37] -> _
    shift-left: _ -> [w38]
    shift-right: [w35] -> _
    shift-left: _ -> [w34]
    tunnel: w8 -> [w33]
    tunnel: w7 -> [w31]
    tunnel: w6 -> [w32]
    tunnel: [w30] -> w5
    tunnel: "second motor T/F" -> [w29]
    tunnel: [w29] -> w2
    stop <- w67 stop-if-true
    # "Std Data"
    # "Std of Sweep"
    # "Mean Data"
    # "Mean of Sweep"
    # "Sweep Number Data"
    # "Grey out Start I/O"
    # "Motor Device Control"
    # "File Path from Export"
    # "Gate Number Data"
    # "Label"
    # "Label"
    # "Label"
    # "Label"
    # "Label"
    # "Label"
    # "Label"
    # "Label"
    # "Label"
    # "Count Data"
    # "RN"
    # "Handle"
    n12 = invoke class="KCubeDCServo" method="GetPositionCounter"(reference=w49) -> ("GetPositionCounter"=w41:i32)  [unwired: 2 in, 2 out]
    n13 = Divide(x=w41, y=1919.6418578623338) -> (x/y=w36:dbl)
    n14 = local write "PC"(w36) -> ()
    n15 = call "SM_CaseSelect.vi"("Input"=w84) -> ("Case"=w85:string)  [unwired: 10 out]
    n16 = case shown="\"MotorJog\"" w85 {
      selector: w85 -> [_ _ _ _ _ _ _ _ _ _ _ _ _ _ _ _ _ _ _ _ _ _ _ _ _ _ w1171 _]
      tunnel: w87 -> [w120 w147 w175 w204 w232 w260 w286 w327 w355 w382 w408 w436 w464 w491 w543 w592 w622 w666 w708 w781 w822 w910 w962 w993 w1049 w1114 w1189 w1214]
      tunnel: [w120 w147 w175 w204 w232 w260 w286 w327 w355 w382 w408 w436 w464 w491 w543 w592 w622 w666 w708 w781 w822 w910 w962 w993 w1049 w1114 w1189 w1214] -> w86
      tunnel: w84 -> [w106 w146 w174 w179 w231 w259 w285 w326 w354 w381 w407 w435 w450 w490 w542 w580 w600 w653 w696 w792 w833 w921 w954 w1006 w1062 w1102 w1188 w1213]
      tunnel: [w105 w146 w174 w179 w231 w259 w285 w326 w354 w381 w407 w435 w449 w490 w542 w579 w599 w654 w697 w792 w833 w921 w953 w1006 w1062 w1099 w1188 w1213] -> w66
      tunnel: w83 -> [_ w134 w162 w192 w219 w247 w273 w313 w341 w369 w396 w423 w452 w479 w531 w581 w611 w656 w698 w791 w832 w920 w974 w1005 w1061 w1113 w1187 w1201]
      tunnel: [w108 w134 w162 w192 w219 w247 w273 w313 w341 w369 w396 w423 w452 w479 w531 w581 w611 w656 w698 w791 w832 w920 w974 w1005 w1061 w1113 w1187 w1201] -> w82
      tunnel: w81 -> [w119 w145 w173 w203 w230 w258 w284 w325 w353 _ w389 w434 w463 w489 w541 w591 w621 w651 w694 w790 w831 w919 w973 w1004 w1060 w1112 w1186 w1212]
      tunnel: [w119 w145 w173 w203 w230 w258 w284 w325 w353 w367 w389 w434 w463 w489 w541 w591 w621 w651 w694 w790 w831 w919 w973 w1004 w1060 w1112 w1186 w1212] -> w80
      tunnel: w79 -> [w118 w144 w172 w202 w229 w257 w283 w324 w352 w380 w406 w433 w462 w478 w527 _ _ w647 w692 w766 w817 w900 w972 w1003 w1059 w1098 w1185 w1211]
      tunnel: [w118 w144 w172 w202 w229 w257 w283 w324 w352 w380 w406 w433 w462 w477 w527 w571 w609 w647 w692 w766 w817 w900 w972 w1003 w1059 w1098 w1185 w1211] -> w78
      tunnel: w77 -> [w117 w143 w171 w201 w228 w256 w282 w323 w351 w379 w405 w432 w461 w488 w540 w590 w620 w665 w707 w789 w830 w918 w970 w1001 w1057 w1111 w1184 w1210]
      tunnel: [w117 w143 w171 w201 w228 w256 w282 w323 w351 w379 w405 w432 w461 w488 w540 w590 w620 w665 w707 w789 w830 w918 w970 w1001 w1057 w1111 w1184 w1210] -> w76
      tunnel: w75 -> [w116 w142 w170 w200 w227 w255 w281 w322 w350 w378 w404 w431 w460 w487 w539 w589 w619 w664 w706 w788 w829 w917 w969 w1000 w1056 w1110 w1183 w1209]
      tunnel: [w116 w142 w170 w200 w227 w255 w281 w322 w350 w378 w404 w431 w460 w487 w539 w589 w619 w664 w706 w788 w829 w917 w969 w1000 w1056 w1110 w1183 w1209] -> w74
      tunnel: w73 -> [w115 w141 w169 w199 w226 w254 w280 w321 w349 w377 w403 w430 w459 w486 w538 w588 w618 w663 w705 w787 w828 w916 w968 w999 w1055 w1109 w1182 w1208]
      tunnel: [w115 w141 w169 w199 w226 w254 w280 w321 w349 w377 w403 w430 w459 w486 w538 w588 w618 w663 w705 w787 w828 w916 w968 w999 w1055 w1109 w1182 w1208] -> w72
      tunnel: w71 -> [w114 w140 w168 w198 w225 w253 w279 w320 w348 w376 w402 w429 w458 w485 w537 w587 w617 w662 w704 w786 w827 w915 w967 w998 w1054 w1108 w1181 w1207]
      tunnel: [w114 w140 w168 w198 w225 w253 w279 w320 w348 w376 w402 w429 w458 w485 w537 w587 w617 w662 w704 w786 w827 w915 w967 w998 w1054 w1108 w1181 w1207] -> w70
      tunnel: w69 -> [w113 w139 w167 w197 w224 w252 w278 w319 w347 w375 w401 w428 w457 w484 w536 w586 w616 w661 w703 w785 w826 w914 w966 w997 w1053 w1107 w1180 w1206]
      tunnel: [w113 w139 w167 w197 w224 w252 w278 w319 w347 w375 w401 w428 w457 w484 w536 w586 w616 w661 w703 w785 w826 w914 w966 w997 w1053 w1107 w1180 w1206] -> w68
      tunnel: [FALSE FALSE FALSE FALSE FALSE FALSE FALSE FALSE FALSE FALSE FALSE FALSE FALSE FALSE FALSE FALSE FALSE FALSE FALSE FALSE FALSE FALSE FALSE FALSE FALSE FALSE FALSE TRUE] -> w67
      tunnel: w64 -> [w109 w135 w163 w193 w220 w248 w274 w315 w343 w371 w397 w424 w453 w480 w532 w582 w612 w657 w699 w784 w825 w913 w965 w996 w1052 w1103 w1176 w1202]
      tunnel: [w109 w135 w163 w193 w220 w248 w274 w315 w343 w371 w397 w424 w453 w480 w532 w582 w612 w657 w699 w784 w825 w913 w965 w996 w1052 w1103 w1176 w1202] -> w63
      tunnel: w62 -> [w111 w137 w165 w195 w222 w250 w276 w317 w345 w373 w399 w426 w455 w482 w534 w584 w614 w659 w701 w783 w824 w912 w964 w995 w1051 w1105 w1178 w1204]
      tunnel: [w111 w137 w165 w195 w222 w250 w276 w317 w345 w373 w399 w426 w455 w482 w534 w584 w614 w659 w701 w783 w824 w912 w964 w995 w1051 w1105 w1178 w1204] -> w61
      tunnel: [w110 w136 w164 w194 w221 w249 w275 w316 w344 w372 w398 w425 w454 w481 w533 w583 w613 w658 w700 w782 w823 w911 w963 w994 w1050 w1104 w1177 w1203] -> w60
      tunnel: w59 -> [w110 w136 w164 w194 w221 w249 w275 w316 w344 w372 w398 w425 w454 w481 w533 w583 w613 w658 w700 w782 w823 w911 w963 w994 w1050 w1104 w1177 w1203]
      tunnel: [w104 w133 w161 w188 w215 w243 w272 w310 w338 w366 w395 w419 w448 w476 w526 w571 w609 w646 w691 w761 w803 w895 w971 w1002 w1058 w1097 w1170 w1200] -> w58
      tunnel: w57 -> [w104 w133 w161 w188 w215 w243 w272 w310 w338 w366 w395 w419 w448 w475 w526 _ _ w646 w691 w761 w803 w895 w971 w1002 w1058 w1097 w1170 w1200]
      tunnel: w56 -> [w103 w132 w160 w187 w214 w242 w271 w309 w337 w365 w394 w418 w447 w474 w530 w570 w608 w645 w690 w763 w815 w897 w961 w992 w1048 w1096 w1169 w1199]
      tunnel: [w103 w132 w160 w187 w214 w242 w271 w309 w337 w365 w394 w418 w447 w474 w530 w570 w608 w645 w690 w763 w815 w897 w961 w992 w1048 w1096 w1169 w1199] -> w55
      tunnel: w54 -> [_ _ _ _ _ _ _ _ _ _ _ _ _ _ _ _ _ _ _ _ _ _ _ w989 w1045 _ _ _]
      tunnel: [w102 w131 w159 w186 w213 w241 w269 w308 w336 w364 w393 w417 w446 w473 w529 w569 w607 w644 w689 w754 w813 w882 w950 w990 w1046 w1095 w1168 w1198] -> w53
      tunnel: w52 -> [w102 w131 w159 w186 w213 w241 w269 w308 w336 w364 w393 w417 w446 w473 w529 w569 w607 w644 w689 w754 w809 w881 _ w990 w1046 w1095 w1168 w1198]
      tunnel: [w101 FALSE FALSE w185 w212 w240 w268 w307 w335 w363 w392 w416 w445 w472 w517 w568 TRUE w643 w688 w756 w812 w894 w959 w988 w1044 w1094 w1167 w1197] -> w51
      tunnel: w50 -> [w101 w130 w158 w185 w212 w240 w268 w307 w335 w363 w392 w416 w445 w472 w517 w568 _ w643 _ w756 w812 w894 w959 w988 w1044 w1094 w1167 w1197]
      tunnel: w48 -> [w99 w127 w155 w184 w211 w239 w267 w306 w334 w362 w387 w415 w444 w471 w528 w567 w605 w642 w687 w755 w808 w891 _ w984 w1043 w1093 w1166 w1196]
      tunnel: [w99 w127 w155 w184 w211 w239 w267 w306 w334 w362 w388 w415 w444 w471 w528 w567 w605 w642 w687 w755 w808 w891 w951 w984 w1043 w1093 w1166 w1196] -> w47
      tunnel: [w98 w126 w154 w183 w210 w238 w266 w305 w333 w361 w391 w414 w443 w470 w518 w566 w604 w641 w684 w753 w811 w886 w958 w986 w1042 w1092 w1165 w1195] -> w46
      tunnel: w45 -> [w98 w126 w154 w183 w210 w238 w266 w305 w333 w361 w391 w414 w443 w470 w518 w566 w604 w641 w684 w753 _ w886 w958 w986 w1042 w1092 w1165 w1195]
      tunnel: [w97 w125 w153 w182 w209 w237 w265 w304 w332 w360 w390 w413 w442 w469 w525 w565 w603 w640 w683 w752 w810 w890 w952 w985 w1041 w1091 w1164 w1194] -> w44
      tunnel: w43 -> [w97 w125 w153 w182 w209 w237 w265 w304 w332 w360 w390 w413 w442 w469 w524 w565 w603 w640 w683 w752 w810 w892 w952 w985 w1041 w1091 w1164 w1194]
      tunnel: w40 -> [w96 w124 w152 w181 w208 w236 w264 w303 w331 w359 w386 w412 w440 w468 w523 w564 w596 w639 w681 w751 w802 w888 w948 w983 w1040 w1090 w1163 w1193]
      tunnel: [w96 w124 w152 w181 w208 w236 w264 w303 w331 w359 w386 w412 w440 w468 w521 w564 w596 w639 w681 w751 w802 w889 w948 w983 w1040 w1090 w1163 w1193] -> w39
      tunnel: w38 -> [w95 w123 w151 w180 w207 w235 w263 w302 w330 w358 w385 w411 w439 w467 w522 w563 w595 w638 w680 w750 _ w885 w947 w982 w1039 w1089 w1162 w1192]
      tunnel: [w95 w123 w151 w180 w207 w235 w263 w302 w330 w358 w385 w411 w439 w467 w522 w563 w595 w638 w680 w750 w801 w885 w947 w982 w1039 w1089 w1162 w1192] -> w37
      tunnel: [w93 w122 w150 w178 w206 w234 w262 w301 w329 w357 w384 w410 w438 w466 w515 w562 w594 w637 w679 w749 w799 w868 w945 w981 w1038 w1088 w1161 w1191] -> w35
      tunnel: w34 -> [w93 w122 w150 w178 w206 w234 w262 w301 w329 w357 w384 w410 w438 w466 w516 w562 w594 w637 w679 w749 w799 _ w945 w981 w1038 w1088 w1161 w1191]
      tunnel: w32 -> [w92 w121 w149 w177 w205 w233 w261 w300 w328 w356 w383 w409 w437 w465 w514 w561 w593 w636 w678 w748 w798 w866 w944 w980 w1037 w1087 w1160 w1190]
      tunnel: w31 -> [_ _ _ _ _ _ _ _ _ _ _ _ _ _ _ _ _ _ _ _ _ _ _ w979 w1034 _ _ _]
      tunnel: [w92 w121 w149 w177 w205 w233 w261 w300 w328 w356 w383 w409 w437 w465 w514 w561 w593 w636 w678 w748 w798 w866 w944 w980 w1037 w1087 w1160 w1190] -> w30
      tunnel: w29 -> [_ _ _ _ _ _ _ _ _ _ _ _ _ _ _ _ _ _ _ _ _ _ _ w976 w1031 _ _ _]
      frame "Initialize" {
        w100 = FALSE ("P1")
        # "Get Device Handle !"
        # "Switch Initialize ....."
        n17 = local write "Export"(w100) -> ()
        n18 = local write "P4"(w100) -> ()
        n19 = local write "P1"(w100) -> ()
        n20 = local write "Start"(w100) -> ()
        n21 = local write "EXIT"(w100) -> ()
        n22 = call "Open.vi"() -> ("Handle Number"=w108:i32)  [unwired: 10 in, 1 out]
        "Handle Number" <- w108
        n23 = local write "P2"(w100) -> ()
        n24 = local write "P5"(w100) -> ()
        n25 = local write "Stop"(w100) -> ()
        n26 = local write "P3"(w100) -> ()
        n27 = local write "P6"(w100) -> ()
        n28 = local write "Auto-Sweep"(w100) -> ()
        n29 = local write "Correction"(TRUE ("P1")) -> ()
        n30 = local write "P7"(w100) -> ()
        n31 = Build Array (concatenate)(w106, "ActiveSwitch") -> (w105:string[])
        n32 = local write "P8"(w100) -> ()
      }
      frame "ActiveSwitch" {
        w128 = T2."Enabled" ("無効")
        # "Set Active Mode to the Switch"
        n33 = property on="P1" class="Bool (strict)"("DisabledEnum"=w128) -> ()  [unwired: 2 in, 2 out]
        n34 = property on="P5" class="Bool (strict)"("DisabledEnum"=w128) -> ()  [unwired: 2 in, 2 out]
        n35 = property on="P7" class="Bool (strict)"("DisabledEnum"=w128) -> ()  [unwired: 2 in, 2 out]
        n36 = property on="P2" class="Bool (strict)"("DisabledEnum"=w128) -> ()  [unwired: 2 in, 2 out]
        n37 = property on="P6" class="Bool (strict)"("DisabledEnum"=w128) -> ()  [unwired: 2 in, 2 out]
        n38 = property on="P8" class="Bool (strict)"("DisabledEnum"=w128) -> ()  [unwired: 2 in, 2 out]
        n39 = property on="P3" class="Bool (strict)"("DisabledEnum"=w128) -> ()  [unwired: 2 in, 2 out]
        n40 = property on="EXIT" class="Bool (strict)"("DisabledEnum"=w128) -> ()  [unwired: 2 in, 2 out]
        n41 = property on="Export" class="Bool (strict)"("DisabledEnum"=w128) -> ()  [unwired: 2 in, 2 out]
        n42 = property on="P4" class="Bool (strict)"("DisabledEnum"=w128) -> ()  [unwired: 2 in, 2 out]
        n43 = case shown="False" w130 {
          tunnel: w128 -> [_ w148]
          frame False {
          }
          frame True {
            n44 = property on="Start" class="Bool (strict)"("DisabledEnum"=w148) -> ()  [unwired: 2 in, 2 out]
          }
        }
      }
      frame "LockSwitch" {
        w156 = T2."Disabled and Grayed Out" ("無効")
        # "Set Lock Mode to the Switch"
        n45 = property on="P1" class="Bool (strict)"("DisabledEnum"=w156) -> ()  [unwired: 2 in, 2 out]
        n46 = property on="P5" class="Bool (strict)"("DisabledEnum"=w156) -> ()  [unwired: 2 in, 2 out]
        n47 = property on="P7" class="Bool (strict)"("DisabledEnum"=w156) -> ()  [unwired: 2 in, 2 out]
        n48 = property on="P2" class="Bool (strict)"("DisabledEnum"=w156) -> ()  [unwired: 2 in, 2 out]
        n49 = property on="P6" class="Bool (strict)"("DisabledEnum"=w156) -> ()  [unwired: 2 in, 2 out]
        n50 = property on="P8" class="Bool (strict)"("DisabledEnum"=w156) -> ()  [unwired: 2 in, 2 out]
        n51 = property on="P3" class="Bool (strict)"("DisabledEnum"=w156) -> ()  [unwired: 2 in, 2 out]
        n52 = property on="EXIT" class="Bool (strict)"("DisabledEnum"=w156) -> ()  [unwired: 2 in, 2 out]
        n53 = property on="Export" class="Bool (strict)"("DisabledEnum"=w156) -> ()  [unwired: 2 in, 2 out]
        n54 = property on="P4" class="Bool (strict)"("DisabledEnum"=w156) -> ()  [unwired: 2 in, 2 out]
        n55 = case shown="False" w158 {
          tunnel: w156 -> [_ w176]
          frame False {
          }
          frame True {
            n56 = property on="Start" class="Bool (strict)"("DisabledEnum"=w176) -> ()  [unwired: 2 in, 2 out]
          }
        }
      }
      frame "SetPower" {
        # "Set power of the PMT-Module"
        n57 = local read "P1"() -> (w191:bool)
        n58 = Boolean To (0,1)(Boolean=w191) -> (0, 1=w190:i16)
        n59 = To Long Integer(number=w190) -> (32bit integer=w189:i32)
        n60 = call "Set HV.vi"("HV"=w189, "handle"=w192) -> ()  [unwired: 8 in, 2 out]
      }
      frame "SetIT" {
        # "Set internal time ....."
        n61 = local read "IT"() -> (w217:i32)
        n62 = To Long Integer(number=w217) -> (32bit integer=w218:i32)
        n63 = call "Set IT.vi"("IT"=w218, "handle"=w219) -> ()  [unwired: 8 in, 2 out]
        n64 = local write "P3"(FALSE ("P3")) -> ()
      }
      frame "SetRN" {
        # "Set read number ....."
        n65 = local read "RN"() -> (w245:i32)
        n66 = To Long Integer(number=w245) -> (32bit integer=w246:i32)
        n67 = call "Set RN.vi"("RN"=w246, "handle"=w247) -> ()  [unwired: 8 in, 2 out]
        n68 = local write "P5"(FALSE ("P3")) -> ()
      }
      frame "SetStepProp" {
        # "Set Step SIze properties....."
        n69 = stacked-sequence {
          frame #0 {
            n70 = local read "WT"() -> (w289:i32)
            n71 = local read "ES"() -> (w288:i32)
            n72 = local read "SS"() -> (w290:i32)
            n73 = local read "EP"() -> (w291:i32)
            n74 = local read "SP"() -> (w292:i32)
            n75 = local write "SSD"(w290) -> ()
            n76 = local write "WTD"(w289) -> ()
            n77 = local write "ESD"(w288) -> ()
            n78 = local write "SPD"(w292) -> ()
            n79 = local write "EPD"(w291) -> ()
            n80 = local read "SP 2"() -> (w287:i32)
            n81 = local write "SPD 2"(w287) -> ()
          }
          frame #1 {
            n82 = local read "SP"() -> (w293:i32)
            n83 = local read "EP"() -> (w295:i32)
            n84 = local read "SS"() -> (w299:i32)
            n85 = local read "ES"() -> (w297:i32)
            n86 = Subtract(x=w295, y=w293) -> (x-y=w294:i32)
            n87 = Divide(x=w294, y=w299) -> (x/y=w298:dbl)
            n88 = Add(x=w298, y=w297) -> (x+y=w296:dbl)
            n89 = local write "SND"(w296) -> ()
          }
        }
        n90 = local write "P7"(FALSE) -> ()
      }
      frame "ReadPower" {
        # "Read power flag of the PMT-Module"
        n91 = local read "PowerD"() -> (w314:i32)
        n92 = call "Read HV.vi"("HV"=w314, "handle"=w313) -> ("HV out"=w312:i32)  [unwired: 7 in, 2 out]
        n93 = local write "PowerD"(w312) -> ()
        n94 = local write "P2"(FALSE ("P2")) -> ()
      }
      frame "ReadIT" {
        # "Read internal time of the PMT-Module"
        n95 = local read "ITD"() -> (w342:i32)
        n96 = call "Read IT.vi"("IT"=w342, "handle"=w341) -> ("IT out"=w340:i32)  [unwired: 7 in, 2 out]
        n97 = local write "ITD"(w340) -> ()
        n98 = local write "P4"(FALSE ("P4")) -> ()
      }
      frame "ReadRN" {
        # "Read data read number of the PMT-Module"
        n99 = local read "RND"() -> (w370:i32)
        n100 = call "Read RN.vi"("RN"=w370, "handle"=w369) -> ("RN out"=w367:i32)  [unwired: 7 in, 2 out]
        n101 = local write "RND"(w367) -> ()
        n102 = local write "P6"(FALSE ("P4")) -> ()
      }
      frame "ReadSN" {
        # "Read data sweep number of the Motorized stage"
        n103 = Increment(x=w387) -> (x+1=w388:i32)
        n104 = local write "SN"(w388) -> ()
      }
      frame "CountStart" {
        # "Conter Start!"
        n105 = local read "Correction"() -> (w420:bool)
        n106 = Boolean To (0,1)(Boolean=w420) -> (0, 1=w422:i16)
        n107 = To Long Integer(number=w422) -> (32bit integer=w421:i32)
        n108 = call "Count Start.vi"("Correction"=w421, "handle"=w423) -> ()  [unwired: 8 in, 2 out]
      }
      frame "CountStop" {
        w441 = FALSE ("Start")
        # "Add Auto Sweep button local variable here"
        # "Conter Stop!"
        n109 = local write "Auto-Sweep"(w441) -> ()
        n110 = local write "Stop"(w441) -> ()
        n111 = local write "Start"(w441) -> ()
        n112 = call "Count Stop.vi"("handle"=w452) -> ()  [unwired: 9 in, 2 out]
        n113 = Build Array (concatenate)(w450, "ActiveSwitch") -> (w449:string[])
      }
      frame "ReadData" {
        # "Read Data...."
        n114 = stacked-sequence {
          seq-local: [_ w500 _] -> [_ _ w510]
          seq-local: [_ w499 _] -> [_ _ w511]
          tunnel: w479 -> [_ w505 _]
          tunnel: w478 -> [_ _ w513]
          tunnel: [_ _ w512] -> w477
          tunnel: [_ w495 _] -> w476
          tunnel: w475 -> [_ w498 _]
          frame #0 {
            # "DB Clear!"
            n115 = Initialize Array(u32 0, 16 ("次元サイズ")) -> (w492:u32[])
            n116 = local write "DB"(w492) -> ()
          }
          frame #1 {
            n117 = local read "OLD"() -> (w502:i32)
            n118 = local read "GN"() -> (w504:i32)
            n119 = local read "DB"() -> (w503:u32[])
            n120 = call "Read Data.vi"("OLD"=w502, "DataBuf"=w503, "GateNum"=w504, "handle"=w505) -> ("OLD out"=w501:i32, "DataBuf out"=w499:u32[], "GateNum out"=w497:i32, "function return"=w500:u32)  [unwired: 3 in, 1 out]
            n121 = local write "OLD"(w501) -> ()
            n122 = local write "GN"(w497) -> ()
            n123 = local write "DB"(w499) -> ()
            n124 = Build Array(w497) -> (w496:i32[])
            n125 = Build Array (concatenate)(w498, w496) -> (w495:i32[])
          }
          frame #2 {
            # "Check Over Rang !"
            # "ADD Data DIM"
            # "Pickup Tans Data!"
            n126 = To Long Integer(number=w510) -> (32bit integer=w508:i32)
            n127 = local read "OLD"() -> (w507:i32)
            n128 = Array Subset(array=w511, length=w508) -> (w509:u32[])  [unwired: 1 in]
            n129 = Not Equal To 0?(x=w507) -> (x != 0?=w506:bool)
            n130 = local write "OVL"(w506) -> ()
            n131 = Build Array (concatenate)(w513, w509) -> (w512:u32[])
            n132 = local write "Graph"(w512) -> ()
          }
        }
      }
      frame "AutoReadData" {
        # "Read Data...."
        n133 = stacked-sequence {
          tunnel: w518 -> [w560]
          tunnel: [w559] -> w525
          tunnel: w524 -> [w554]
          tunnel: w523 -> [w558]
          tunnel: w522 -> [w557]
          tunnel: [w556] -> w521
          tunnel: w518 -> [w555]
          tunnel: w516 -> [w549]
          tunnel: [w547] -> w515
          frame #0 {
            n134 = local read "SP"() -> (w551:i32)
            n135 = local read "SS"() -> (w546:i32)
            n136 = Array Size(array=w554) -> (size(s)=w553:i32)
            n137 = Multiply(x=w546, y=2) -> (x*y=w545:i32)
            n138 = Multiply(x=w545, y=w553) -> (x*y=w552:i32)
            n139 = Add(x=w551, y=w552) -> (x+y=w550:i32)
            n140 = Bundle("mean"=w555, w550) -> (w548:cluster{"mean":dbl, i32})  [unwired: 1 in]
            n141 = Build Array (concatenate)(w558, w557) -> (w556:dbl[])
            n142 = Build Array (concatenate)(w554, w560) -> (w559:dbl[])
            n143 = Build Array (concatenate)(w549, w548) -> (w547:cluster{"mean":dbl, i32}[])
            n144 = local write "Sweep Graph"(w559) -> ()
          }
        }
        n145 = property on="Polar Plot" class="Pict"() -> ("Draw Area Size"=w520:T3)  [unwired: 2 in, 2 out]
        n146 = call <vilib>:"Polar Plot with Point Options.vi"("data array [mag, phase (deg)]"=w515, "dimensions (w,h)"=w520) -> ("new picture"=→"Polar Plot":picture)  [unwired: 13 in]
      }
      frame "CountInit" {
        w573 = 0
        # "Auto"
        # "Clear Data DIM !"
        n147 = Initialize Array(w573, w573) -> (w571:i32[])
        n148 = Build Array("LockSwitch", "ReadRN", "CountStart", "ReadData", "CheckNumber") -> (w574:string[])
        n149 = Build Array (concatenate)(w580, w574) -> (w579:string[])
      }
      frame "AutoCount|nit!" {
        w610 = 0
        # "Clear Data DIM !"
        n150 = local read "SND"() -> (w597:i32)
        n151 = local read "SN"() -> (w602:i32)
        n152 = Increment(x=w597) -> (x+1=w598:i32)
        n153 = Initialize Array(w610, w610) -> (w609:i32[])
        n154 = Less?(x=w602, y=w598) -> (x < y?=w601:bool)
        n155 = case shown="True" w601 {
          tunnel: w600 -> [w626 w629]
          tunnel: [w624 w628] -> w599
          frame False {
            n156 = Build Array("AutoReadData", "AutoCheckNumber") -> (w625:string[])
            n157 = Build Array (concatenate)(w626, w625) -> (w624:string[])
          }
          frame True {
            n158 = Build Array("LockSwitch", "ReadRN", "CountStart", "ReadData", "AutoCheckNumber") -> (w635:string[])
            n159 = Build Array (concatenate)(w629, w635) -> (w628:string[])
          }
        }
      }
      frame "CheckNumber" {
        # "Add append"
        # "Add Case Strucutre outside\nsimilar to GN,"
        # "Check RN and Data lenbgth,Stop Switch ......"
        n160 = local read "Stop"() -> (w648:bool)
        n161 = local read "GN"() -> (w649:i32)
        n162 = Decrement(x=w651) -> (x-1=w650:i32)
        n163 = Less?(x=w649, y=w650) -> (x < y?=w655:bool)
        n164 = case shown="True" w655 {
          tunnel: [w670 w672] -> w652
          tunnel: w648 -> [_ w671]
          frame False {
            # "\"MotorJog\"; here"
            # "Move \"Active Swith\" to False Condition of Position Number"
            # "Add \"AutoExport Run\" here"
            n165 = local write "Start"(FALSE ("Start")) -> ()
            n166 = Build Array("CountStop", "ActiveSwitch") -> (w670:string[])
          }
          frame True {
            n167 = case shown="True" w671 {
              tunnel: [w674 w676] -> w672
              frame False {
                n168 = Build Array("ReadData", "CheckNumber") -> (w674:string[])
              }
              frame True {
                n169 = Build Array("CountStop") -> (w676:string[])
              }
            }
          }
        }
        n170 = Build Array (concatenate)(w653, w652) -> (w654:string[])
      }
      frame "AutoCheckNumber" {
        # "Add append"
        # "Add Case Strucutre outside\nsimilar to GN,"
        # "Check RN and Data lenbgth,Stop Switch ......"
        n171 = local read "Stop"() -> (w693:bool)
        n172 = local read "SND"() -> (w682:i32)
        n173 = local read "SN"() -> (w686:i32)
        n174 = Less?(x=w686, y=w682) -> (x < y?=w685:bool)
        n175 = case shown="False" w685 {
          tunnel: [w710 w720] -> w695
          tunnel: w694 -> [_ w719]
          tunnel: w693 -> [_ w716]
          tunnel: [TRUE w715] -> w688
          frame False {
            w714 = FALSE ("Start")
            n176 = local write "Auto-Sweep"(w714) -> ()
            n177 = local write "Start"(w714) -> ()
            n178 = Build Array("CountStop", "AutoExportSweep", "ActiveSwitch") -> (w710:string[])
          }
          frame True {
            n179 = local read "GN"() -> (w717:i32)
            n180 = Decrement(x=w719) -> (x-1=w718:i32)
            n181 = Less?(x=w717, y=w718) -> (x < y?=w721:bool)
            n182 = case shown="False" w721 {
              tunnel: [w723 w739] -> w720
              tunnel: w716 -> [w724 w738]
              tunnel: [w722 w737] -> w715
              frame False {
                # "\"MotorJog\"; here"
                # "Move \"Active Swith\" to False Condition of Position Number"
                # "Add \"AutoExport Run\" here"
                n183 = case shown="False" w724 {
                  tunnel: [w730 w735] -> w723
                  tunnel: [FALSE TRUE] -> w722
                  frame False {
                    n184 = Build Array("CountStop", "AutoExportRun", "AutoReadData", "ReadSN", "MotorJog", "AutoCount|nit!") -> (w730:string[])
                  }
                  frame True {
                    n185 = local write "Auto-Sweep"(TRUE) -> ()
                    n186 = Build Array("CountStop") -> (w735:string[])
                  }
                }
              }
              frame True {
                n187 = case shown="False" w738 {
                  tunnel: [w742 w746] -> w739
                  tunnel: [FALSE TRUE] -> w737
                  frame False {
                    n188 = Build Array("ReadData", "AutoCheckNumber") -> (w742:string[])
                  }
                  frame True {
                    n189 = Build Array("CountStop") -> (w746:string[])
                    n190 = local write "Auto-Sweep"(TRUE) -> ()
                  }
                }
              }
            }
          }
        }
        n191 = Build Array (concatenate)(w696, w695) -> (w697:string[])
      }
      frame "Export" {
        # "For Auto Export also add mean waveform"
        # "Get mean Data into 1D array Shift register for waveform"
        # "Gate Number is just number of count measurements"
        # "time...using array size"
        # "time...using array size"
        n192 = Array Size(array=w766) -> (size(s)=w778:i32)
        n193 = for {
          N: w778 -> [_]
          tunnel: [w793] -> w765 mode=indexing
          i -> [w795]
          n194 = local read "ITD"() -> (w797:i32)
          n195 = Add(x=1, y=w795) -> (x+y=w796:i32)
          n196 = Multiply(x=w797, y=w796) -> (x*y=w793:i32)
        }
        n197 = call <vilib>:"Std Deviation and Variance.vi"("X"=w766) -> ("mean"=w759:dbl, "standard deviation"=w758:dbl)  [unwired: 1 in, 1 out]
        n198 = Build Array(w759, w758) -> (w757:dbl[])
        n199 = Build Array(w761, w765, w766) -> (w776:u32[][])
        n200 = call-poly <vilib>:"Write Delimited Spreadsheet.vi"("1D data"=string[] ["Gate  No.", "Time [ms]", "Counts"], "append to file? (new file:F)"=FALSE, "transpose? (no:F)"=FALSE) -> ("new file path (Not A Path if cancelled)"=w775:path)  [unwired: 11 in, 1 out]
        n201 = call-poly <vilib>:"Write Delimited Spreadsheet.vi"("file path (dialog if empty)"=w775, "2D data"=w776, "append to file? (new file:F)"=TRUE, "transpose? (no:F)"=TRUE) -> ("new file path (Not A Path if cancelled)"=w771:path)  [unwired: 10 in, 1 out]
        n202 = call-poly <vilib>:"Write Delimited Spreadsheet.vi"("file path (dialog if empty)"=w771, "1D data"=string[] ["Mean", "Std. Dev."], "append to file? (new file:F)"=TRUE, "transpose? (no:F)"=FALSE) -> ("new file path (Not A Path if cancelled)"=w767:path)  [unwired: 10 in, 1 out]
        n203 = call-poly <vilib>:"Write Delimited Spreadsheet.vi"("file path (dialog if empty)"=w767, "1D data"=w757, "append to file? (new file:F)"=TRUE, "transpose? (no:F)"=FALSE) -> ()  [unwired: 10 in, 2 out]
        n204 = local write "Export"(FALSE) -> ()
      }
      frame "AutoExportRun" {
        # "For Auto Export also add mean waveform"
        # "Get mean Data into 1D array Shift register for waveform"
        # "Gate Number is just number of count measurements"
        # "time...using array size"
        n205 = Array Size(array=w817) -> (size(s)=w819:i32)
        n206 = for {
          N: w819 -> [_]
          tunnel: [w861] -> w816 mode=indexing
          i -> [w863]
          n207 = local read "ITD"() -> (w865:i32)
          n208 = Add(x=1, y=w863) -> (x+y=w864:i32)
          n209 = Multiply(x=w865, y=w864) -> (x*y=w861:i32)
        }
        n210 = flat-sequence {
          tunnel: w808 -> [w860]
          tunnel: [w856] -> w807
          frame #0 {
            n211 = local read "SS"() -> (w859:i32)
            n212 = Multiply(x=w860, y=w859) -> (x*y=w857:i32)
            n213 = local read "SP"() -> (w858:i32)
            n214 = Add(x=w858, y=w857) -> (x+y=w856:i32)
          }
        }
        n215 = call <vilib>:"Std Deviation and Variance.vi"("X"=w817) -> ("mean"=w811:dbl, "standard deviation"=w801:dbl)  [unwired: 1 in, 1 out]
        n216 = Build Array(w811, w801) -> (w814:dbl[])
        n217 = Number To Decimal String(number=w807) -> (decimal integer string=w806:string)  [unwired: 1 in]
        n218 = Build Array(w803, w816, w817) -> (w818:u32[][])
        n219 = Build Array (concatenate)(string[] ["Angle (deg)"], w806) -> (w804:string[])
        n220 = case shown="True" "Save All Gate Data" {
          tunnel: w818 -> [_ w854]
          tunnel: w814 -> [_ w841]
          tunnel: [w834 w840] -> w813
          tunnel: w809 -> [w834 w839]
          tunnel: w804 -> [_ w835]
          frame False {
          }
          frame True {
            # "time...using array size"
            n221 = call-poly <vilib>:"Write Delimited Spreadsheet.vi"("file path (dialog if empty)"=w839, "1D data"=w835, "append to file? (new file:F)"=TRUE, "transpose? (no:F)"=FALSE) -> ("new file path (Not A Path if cancelled)"=w838:path)  [unwired: 10 in, 1 out]
            n222 = call-poly <vilib>:"Write Delimited Spreadsheet.vi"("file path (dialog if empty)"=w838, "1D data"=string[] ["Gate  No.", "Time [ms]", "Counts"], "append to file? (new file:F)"=TRUE, "transpose? (no:F)"=FALSE) -> ("new file path (Not A Path if cancelled)"=w853:path)  [unwired: 10 in, 1 out]
            n223 = call-poly <vilib>:"Write Delimited Spreadsheet.vi"("file path (dialog if empty)"=w853, "2D data"=w854, "append to file? (new file:F)"=TRUE, "transpose? (no:F)"=TRUE) -> ("new file path (Not A Path if cancelled)"=w849:path)  [unwired: 10 in, 1 out]
            n224 = call-poly <vilib>:"Write Delimited Spreadsheet.vi"("file path (dialog if empty)"=w849, "1D data"=string[] ["Mean", "Std. Dev."], "append to file? (new file:F)"=TRUE, "transpose? (no:F)"=FALSE) -> ("new file path (Not A Path if cancelled)"=w845:path)  [unwired: 10 in, 1 out]
            n225 = call-poly <vilib>:"Write Delimited Spreadsheet.vi"("file path (dialog if empty)"=w845, "1D data"=w841, "append to file? (new file:F)"=TRUE, "transpose? (no:F)"=FALSE) -> ("new file path (Not A Path if cancelled)"=w840:path)  [unwired: 10 in, 1 out]
          }
        }
        n226 = local write "Export"(FALSE) -> ()
      }
      frame "AutoExportSweep" {
        w870 = 0
        w869 = 0.0
        # "Gate Number is just number \nof count measurements"
        # "For Auto Export also add mean waveform"
        # "Get mean Data into 1D array Shift register for waveform"
        # "time...using array size"
        # "time...using array size"
        n227 = Array Size(array=w892) -> (size(s)=w907:i32)
        n228 = for {
          N: w907 -> [_]
          tunnel: [w942] -> w899 mode=indexing
          i -> [w939]
          n229 = local read "SS"() -> (w943:i32)
          n230 = Multiply(x=w943, y=w939) -> (x*y=w940:i32)
          n231 = local read "SP"() -> (w941:i32)
          n232 = Add(x=w941, y=w940) -> (x+y=w942:i32)
        }
        n233 = call <vilib>:"Std Deviation and Variance.vi"("X"=w892) -> ("mean"=w893:dbl, "standard deviation"=w887:dbl)  [unwired: 1 in, 1 out]
        n234 = Initialize Array(w869, w870) -> (w890:dbl[])
        n235 = Initialize Array(w869, w870) -> (w889:dbl[])
        n236 = Build Array(w893, w887) -> (w883:dbl[])
        n237 = Initialize Array(cluster{i32, i32} {0, 0}, w870) -> (w868:cluster{i32, i32}[])
        n238 = Build Array(w899, w892, w888) -> (w905:dbl[][])
        n239 = local read "RN"() -> (w875:i32)
        n240 = Number To Decimal String(number=w875) -> (decimal integer string=w874:string)  [unwired: 1 in]
        n241 = local read "IT"() -> (w873:i32)
        n242 = Number To Decimal String(number=w873) -> (decimal integer string=w872:string)  [unwired: 1 in]
        n243 = Build Array("Sample Name", "Laser Power (mW)", w874, w872) -> (w871:string[])
        n244 = for {
          N: 4 -> [_]
          shift-right: [w927] -> w878
          shift-left: w881 -> [w928]
          tunnel: string[] ["#Sample", "#LaserPower (mW)", "#NumGates", "#GateTime (ms)"] -> [w923] mode=indexing
          tunnel: w871 -> [w922] mode=indexing
          n245 = Build Array(w923, w922) -> (w924:string[])
          n246 = call-poly <vilib>:"Write Delimited Spreadsheet.vi"("file path (dialog if empty)"=w928, "1D data"=w924, "append to file? (new file:F)"=TRUE, "transpose? (no:F)"=FALSE) -> ("new file path (Not A Path if cancelled)"=w927:path)  [unwired: 10 in, 1 out]
        }
        n247 = call-poly <vilib>:"Write Delimited Spreadsheet.vi"("file path (dialog if empty)"=w878, "1D data"=string[] ["Angle", "CountsMean", "CountsSTD"], "append to file? (new file:F)"=TRUE, "transpose? (no:F)"=FALSE) -> ("new file path (Not A Path if cancelled)"=w904:path)  [unwired: 10 in, 1 out]
        n248 = call-poly <vilib>:"Write Delimited Spreadsheet.vi"("file path (dialog if empty)"=w904, "2D data"=w905, "append to file? (new file:F)"=TRUE, "transpose? (no:F)"=TRUE) -> ("new file path (Not A Path if cancelled)"=w901:path)  [unwired: 10 in, 1 out]
        n249 = case shown="False" FALSE {
          tunnel: w901 -> [w929 w937]
          tunnel: w883 -> [_ w934]
          tunnel: [w929 w931] -> w882
          frame False {
          }
          frame True {
            n250 = call-poly <vilib>:"Write Delimited Spreadsheet.vi"("file path (dialog if empty)"=w937, "1D data"=string[] ["Mean", "Std. Dev."], "append to file? (new file:F)"=TRUE, "transpose? (no:F)"=FALSE) -> ("new file path (Not A Path if cancelled)"=w935:path)  [unwired: 10 in, 1 out]
            n251 = call-poly <vilib>:"Write Delimited Spreadsheet.vi"("file path (dialog if empty)"=w935, "1D data"=w934, "append to file? (new file:F)"=TRUE, "transpose? (no:F)"=FALSE) -> ("new file path (Not A Path if cancelled)"=w931:path)  [unwired: 10 in, 1 out]
          }
        }
        n252 = local write "Export"(FALSE) -> ()
      }
      frame "AutoSweep" {
        w951 = 0
        # "1. Create a file path (Send two strings, \"SetPosition\" and \"AutoCount|nit!\")\n2. Send to \"SetPosition\"\n2.1. Will create a Position Number Shift register\n2.2. Move stage to initial position, allow time to complete movement or add delay\n3. Send to \"AutoCount|nit!\"\n3.1. \"AutoCount|nit!\" is clone of \"Count|nit!\" but sends to \"AutoCheckNumber\", not \"CheckNumber\n3.1.1. \"AutoCheckNumber\" will check if end position, or run condition is met then send \"CountStop\" and \"ActiveSwitch\"\n3.1.2. \"AutoCheck Number\" will allow \"CountStop\" to be sent via Stop Boolean\n3.1.3. \"AutoCheckNumber\" will upon END of one run will run \"AutoExportRun\" to set file path\n3.1.3.1. \"AutoExportRun\" will add a data point to Mean Waveform after Count Stop\n3.1.4. \"AutoCheckNumber\" will upon END of sweep will run \"AutoExportSweep\" then issue \"ActiveSwitch\"\n3.1.4.1. \"AutoExportSweep\" will append final Mean Sweep waveform to file path before \"CountStop\";\"ActiveSwitch\"\n4. If End condition not met; \"MotorJog\"; \"AutoCount|nit!\"....repeats\n4.1. Will move to next position by set increment, with .net code, add delay to allow it to arrive at position"
        # "Create a File path here\nSend switch case string \"SetPosition\", which has a position number switch register"
        # "1.Position Set, create a file path\n2. Count|nit!---duplicate and create auto counter, add read sweep data for auto read\n2.0.1Checknumber end, change active switch to Auto export\n3. Auto Export ... need to make \n3.0.2Auto Export end, send to read sweep data (mean, stdev for per sweep)\n3.Export\n4.check end position, check end condition met\n5.met>end;not end >continue\n6. Jog motor\n7.repeat from 2."
        # "Create Motor Controls for setting Homing, Step size for angle, idle time(if required),"
        n253 = local write "SN"(w951) -> ()
        n254 = call-poly <vilib>:"Write Delimited Spreadsheet.vi"("append to file? (new file:F)"=FALSE) -> ("new file path (Not A Path if cancelled)"=w950:path)  [unwired: 13 in, 1 out]
        n255 = Build Array("SetPosition", "AutoCount|nit!") -> (w956:string[])
        n256 = Build Array (concatenate)(w954, w956) -> (w953:string[])
        n257 = Wait (ms)(milliseconds to wait="Wait to Start (ms)") -> ()  [unwired: 1 out]
      }
      frame "MotorJog" {
        # "Move position by set increment"
        # "Add a test Jog?"
        # "Put thor labs net code here"
        n258 = flat-sequence {
          tunnel: w989 -> [w1013]
          tunnel: [w1013] -> w978
          tunnel: w979 -> [w1008]
          tunnel: [w1008] -> w977
          tunnel: w976 -> [w1007]
          tunnel: [w1007] -> w975
          tunnel: w978 -> [w1026]
          tunnel: w977 -> [w1021]
          tunnel: w975 -> [w1020]
          frame #0 {
            n259 = case shown="True" w1007 {
              tunnel: w1008 -> [_ w1017]
              frame False {
              }
              frame True {
                n260 = local read "SSD"() -> (w1015:i32)
                n261 = Multiply(x=w1015, y=2) -> (x*y=w1016:i32)
                n262 = invoke class="KCubeDCServo" method="MoveRelative"(reference=w1017, "direction"=1, "stepSize"=w1016, "waitTimeout"=0) -> ()  [unwired: 2 in, 6 out]
              }
            }
            n263 = local read "SSD"() -> (w1012:i32)
            n264 = invoke class="KCubeDCServo" method="MoveRelative"(reference=w1013, "direction"=1, "stepSize"=w1012, "waitTimeout"=0) -> ()  [unwired: 2 in, 6 out]
            n265 = local read "WT"() -> (w1010:i32)
            n266 = Wait (ms)(milliseconds to wait=w1010) -> ()  [unwired: 1 out]
          }
          frame #1 {
            n267 = case shown="True" w1020 {
              tunnel: w1021 -> [_ w1027]
              frame False {
              }
              frame True {
                n268 = invoke class="KCubeDCServo" method="GetPositionCounter"(reference=w1027) -> ("GetPositionCounter"=w1030:i32)  [unwired: 2 in, 2 out]
                n269 = Divide(x=w1030, y=1919.6418578623338) -> (x/y=w1028:dbl)
                n270 = local write "PC 2"(w1028) -> ()
              }
            }
            n271 = invoke class="KCubeDCServo" method="GetPositionCounter"(reference=w1026) -> ("GetPositionCounter"=w1024:i32)  [unwired: 2 in, 2 out]
            n272 = Divide(x=w1024, y=1919.6418578623338) -> (x/y=w1022:dbl)
            n273 = local write "PC"(w1022) -> ()
            n274 = Wait (ms)(milliseconds to wait=50) -> ()  [unwired: 1 out]
          }
        }
        n275 = local write "P8"(FALSE) -> ()
      }
      frame "SetPosition" {
        n276 = flat-sequence {
          tunnel: w1045 -> [w1066]
          tunnel: [w1066] -> w1036
          tunnel: w1034 -> [w1064]
          tunnel: [w1064] -> w1033
          tunnel: w1031 -> [w1063]
          tunnel: w1036 -> [w1073]
          tunnel: [w1073] -> w1035
          tunnel: w1033 -> [w1071]
          tunnel: [w1071] -> w1032
          tunnel: w1031 -> [w1069]
          tunnel: w1035 -> [w1082]
          tunnel: w1032 -> [w1077]
          tunnel: w1031 -> [w1076]
          frame #0 {
            n277 = case shown="True" w1063 {
              tunnel: w1064 -> [_ w1068]
              frame False {
              }
              frame True {
                n278 = local read "SPD 2"() -> (w1067:i32)
                n279 = invoke class="KCubeDCServo" method="SetMoveAbsolutePosition"(reference=w1068, "position"=w1067) -> ()  [unwired: 2 in, 4 out]
              }
            }
            n280 = local read "SPD"() -> (w1065:i32)
            n281 = invoke class="KCubeDCServo" method="SetMoveAbsolutePosition"(reference=w1066, "position"=w1065) -> ()  [unwired: 2 in, 4 out]
          }
          frame #1 {
            w1070 = 0
            n282 = case shown="True" w1069 {
              tunnel: w1071 -> [_ w1075]
              tunnel: w1070 -> [_ w1074]
              frame False {
              }
              frame True {
                n283 = invoke class="KCubeDCServo" method="MoveAbsolute"(reference=w1075, "waitTimeout"=w1074) -> ()  [unwired: 2 in, 4 out]
              }
            }
            n284 = invoke class="KCubeDCServo" method="MoveAbsolute"(reference=w1073, "waitTimeout"=w1070) -> ()  [unwired: 2 in, 4 out]
            n285 = local read "WT"() -> (w1072:i32)
            n286 = Wait (ms)(milliseconds to wait=w1072) -> ()  [unwired: 1 out]
          }
          frame #2 {
            n287 = case shown="True" w1076 {
              tunnel: w1077 -> [_ w1084]
              frame False {
              }
              frame True {
                n288 = invoke class="KCubeDCServo" method="GetPositionCounter"(reference=w1084) -> ("GetPositionCounter"=w1085:i32)  [unwired: 2 in, 2 out]
                n289 = Divide(x=w1085, y=1919.6418578623338) -> (x/y=w1083:dbl)
                n290 = local write "PC 2"(w1083) -> ()
              }
            }
            n291 = invoke class="KCubeDCServo" method="GetPositionCounter"(reference=w1082) -> ("GetPositionCounter"=w1079:i32)  [unwired: 2 in, 2 out]
            n292 = Divide(x=w1079, y=1919.6418578623338) -> (x/y=w1078:dbl)
            n293 = local write "PC"(w1078) -> ()
            n294 = Wait (ms)(milliseconds to wait=50) -> ()  [unwired: 1 out]
          }
        }
      }
      frame "", "Idle" {
        n295 = event shown="[12] \"Auto-Sweep\": Value Change" {
          selector: _ -> [_ _ _ _ _ _ _ _ _ _ _ _ _]
          dyn-events: _ -> [_ _ _ _ _ _ _ _ _ _ _ _ _]
          timeout: _ -> [_ _ _ _ _ _ _ _ _ _ _ _ _]
          tunnel: w1102 -> [w1117 w1120 w1123 w1127 w1131 w1135 w1139 w1143 w1146 w1148 w1151 w1154 w1157]
          tunnel: [w1115 w1119 w1122 w1126 w1130 w1134 w1138 w1142 w1145 w1147 w1150 w1153 w1158] -> w1100
          event Menu Selection (User) {
            n296 = event-data() -> ("ItemTag"=w1116:string)  [unwired: 1 out]
            n297 = Build Array (concatenate)(w1117, w1116) -> (w1115:string[])
          }
          event "EXIT": Value Change {
            n298 = event-data() -> ()  [unwired: 7 out]
            n299 = Build Array (concatenate)(w1120, "Exit") -> (w1119:string[])
          }
          event "P1": Value Change {
            n300 = event-data() -> ()  [unwired: 7 out]
            n301 = Build Array (concatenate)(w1123, "SetPower") -> (w1122:string[])
          }
          event "P2": Value Change {
            n302 = event-data() -> ()  [unwired: 7 out]
            n303 = Build Array (concatenate)(w1127, "ReadPower") -> (w1126:string[])
            n304 = Wait (ms)(milliseconds to wait=u32 200 ("ミリ秒待機時間")) -> ()  [unwired: 1 out]
          }
          event "P3": Value Change {
            n305 = event-data() -> ()  [unwired: 7 out]
            n306 = Build Array (concatenate)(w1131, "SetIT") -> (w1130:string[])
            n307 = Wait (ms)(milliseconds to wait=u32 200 ("ミリ秒待機時間")) -> ()  [unwired: 1 out]
          }
          event "P4": Value Change {
            n308 = event-data() -> ()  [unwired: 7 out]
            n309 = Build Array (concatenate)(w1135, "ReadIT") -> (w1134:string[])
            n310 = Wait (ms)(milliseconds to wait=u32 200 ("ミリ秒待機時間")) -> ()  [unwired: 1 out]
          }
          event "P5": Value Change {
            n311 = event-data() -> ()  [unwired: 7 out]
            n312 = Build Array (concatenate)(w1139, "SetRN") -> (w1138:string[])
            n313 = Wait (ms)(milliseconds to wait=u32 200 ("ミリ秒待機時間")) -> ()  [unwired: 1 out]
          }
          event "P6": Value Change {
            n314 = event-data() -> ()  [unwired: 7 out]
            n315 = Build Array (concatenate)(w1143, "ReadRN") -> (w1142:string[])
            n316 = Wait (ms)(milliseconds to wait=u32 200 ("ミリ秒待機時間")) -> ()  [unwired: 1 out]
          }
          event "Start": Value Change {
            n317 = event-data() -> ()  [unwired: 7 out]
            n318 = Build Array (concatenate)(w1146, "CountInit") -> (w1145:string[])
          }
          event "Export": Value Change {
            n319 = event-data() -> ()  [unwired: 7 out]
            n320 = Build Array (concatenate)(w1148, "Export") -> (w1147:string[])
          }
          event "P7": Value Change {
            n321 = event-data() -> ()  [unwired: 7 out]
            n322 = Build Array (concatenate)(w1151, "SetStepProp") -> (w1150:string[])
          }
          event "P8": Value Change {
            n323 = event-data() -> ()  [unwired: 7 out]
            n324 = Build Array (concatenate)(w1154, "MotorJog") -> (w1153:string[])
          }
          event "Auto-Sweep": Value Change {
            n325 = event-data() -> ()  [unwired: 7 out]
            n326 = Build Array (concatenate)(w1157, "AutoSweep") -> (w1158:string[])
            n327 = Wait (ms)(milliseconds to wait=200) -> ()  [unwired: 1 out]
          }
        }
        n328 = Build Array (concatenate)("", w1100) -> (w1099:string[])
      }
      frame "Error", Default {
        n329 = Concatenate Strings("Error  Case Name .....", "\r\n", w1171) -> (w1173:string)
        n330 = One Button Dialog(message=w1173) -> (true=w1172:bool)  [unwired: 1 out]
        n331 = stacked-sequence {
          tunnel: w1172 -> [_]
          frame #0 {
            n332 = Stop() -> ()  [unwired: 1 out]
          }
        }
      }
      frame "Exit" {
        # "See you again ......"
        n333 = call "Close.vi"("Handle"=w1201) -> ()  [unwired: 9 in, 2 out]
      }
    }
    n334 = case shown="True" w29 {
      tunnel: w33 -> [_ w88]
      frame False {
      }
      frame True {
        n335 = invoke class="KCubeDCServo" method="GetPositionCounter"(reference=w88) -> ("GetPositionCounter"=w90:i32)  [unwired: 2 in, 2 out]
        n336 = Divide(x=w90, y=1919.6418578623338) -> (x/y=w89:dbl)
        n337 = local write "PC 2"(w89) -> ()
      }
    }
    n338 = call "SM_CaseErase.vi"("Input"=w66) -> ("Output"=w65:string[])  [unwired: 10 out]
  }
  n339 = case shown="True" w2 {
    tunnel: w5 -> [_ w1215]
    frame False {
    }
    frame True {
      n340 = invoke class="KCubeDCServoControl" method="CloseDevice"(reference=w1215) -> ()  [unwired: 2 in, 3 out]
    }
  }
  n341 = invoke class="KCubeDCServoControl" method="CloseDevice"(reference=w13) -> ()  [unwired: 2 in, 3 out]
